vi "Main - 17JuneBackup.vi"() -> ()   [LabVIEW 2018]
uses:
  LoadCellType.ctl
  MotorUnits.ctl
  CalibrationComponentsList.ctl
  CalibrationValuesList.ctl
  CalibrationFileHeaders.ctl
  <vilib>/Analysis/baseanly.llb/Mean (DBL).vi
  1bae0f2e-106e-414f-9c47-dad4a1d3b324.vi
  c2e41f69-c736-4862-8fa9-ab2912e2b40f.vi
  8906c7f1-8855-440d-adf6-1dafab09265a.vi
  e867b6df-3684-438a-bb7f-c804a2c90fcb.vi
  489dc40e-59c5-4e85-922b-f9ff9f858a38.vi
  441b7fa7-1fda-4f0d-8a96-d35181be4240.vi
  76a06f91-e74a-4c68-b1da-59c59035c8f1.vi
  95c3a942-58a8-4429-8ed6-39484f079eb5.vi
  aa792640-a713-44b5-b5bc-ea87e5fc700a.vi
  <vilib>/Utility/file.llb/Write Delimited Spreadsheet (string).vi
  <vilib>/Utility/file.llb/Read Delimited Spreadsheet (string).vi
  <vilib>/FPGAPlugInAG/myRIO-1900/niLvFpga_Open_myRIO-1900.vi
  <vilib>/rvi/interface/common/dynamic/niFpgaDynamicAddResources.vi
  <vilib>/FPGAPlugInAG/Dynamic/niLvFpga_Run_Dynamic.vi
  <vilib>/Utility/error.llb/Error Cluster From Error Code.vi
  <vilib>/rvi/errors/niLvFpgaAdjustHostInterfaceError.vi
  <vilib>/FPGAPlugInAG/Dynamic/niLvFpga_Abort_Dynamic.vi
  <vilib>/FPGAPlugInAG/Dynamic/niLvFpga_Close_Dynamic.vi
  <vilib>/Utility/file.llb/Write Delimited Spreadsheet (DBL).vi
  <vilib>/rvi/interface/nirviOpenFPGA/nirviOpenFPGA.xnode
  FPGA Bitfiles/StandProgram_FPGATarget2_FPGALeftReadout2_EZoqyqWkBrw.lvbitx
  FPGALeftReadout.vi
  <vilib>/rvi/interface/nirviMethod/nirviMethod.xnode
  FPGA Bitfiles/StandProgram_FPGATarget3_FPGARightReadout_3OIjwdsUrXE.lvbitx
  FPGARightReadout.vi
  <vilib>/rvi/interface/nirviReadWriteControl/nirviReadWriteControl.xnode
  <vilib>/rvi/interface/nirviCloseFPGA/nirviCloseFPGA.xnode
  FPGA Bitfiles/StandProgram_FPGATarget_FPGACentreReadou_28m02jle5Aw.lvbitx
  FPGACentreReadout.vi
  NiFpgaLv.dll
  <vilib>/rvi/interface/Simulation/niFpgaSimulationCallBeginRW.vi
  <vilib>/Analysis/NI_AALBase.lvlib
  <userlib>/dxl_x86_c/dxl_x86_c.lvlib
panel:
  out "Torque Timer [s]":dbl
  out "Thrust Timer [s]":dbl
  out "Torque PID out":dbl
  out "Thrust PID out":dbl
  out "Torque error_i":dbl
  out "Torque error_last":dbl
  out "Torque error_d":dbl(graph)
  out "Thrust error_d":dbl(graph)
  out "Thrust error_i":dbl
  out "Thrust error_last":dbl
  in  "PID Min":dbl=60.0 format="%#_13g"
  out "Time under tolerance":dbl
  in  "Torque tolerance [Nm]":dbl=0.01 step=0.001
  in  "Thrust tolerance [g]":dbl=3.0 step=0.1
  out "Torque error [Nm]":dbl
  out "Thrust error [g]":dbl
  in  "Torque Collum":dbl=5.0
  in  "Torque Row":dbl=2.0
  in  "Thrust Collum":dbl=4.0
  in  "Thrust Row":dbl=2.0
  in  "Setlting time [s]":i32=5
  out "Total Torque":dbl(graph)
  out "Total Thrust":dbl(graph)
  in  "PID Max":dbl=1000.0 format="%#_13g"
  in  "kp_m":dbl step=1.0
  in  "ki_m":dbl step=1.0
  in  "kd_m":dbl step=0.1
  in  "kd_t":dbl step=0.1
  in  "ki_t":dbl=0.25 step=0.001
  in  "kp_t":dbl=0.10000000000000003 step=0.1
  out "Closed Loop Left output":dbl
  out "Closed Loop Right output":dbl
  in  "Closed loop":bool
  in  "Total Desired Torque [Nm]":dbl step=0.01
  in  "Total Desired Thrust [g]":dbl step=50.0
  out "Dxl 2 Pos":dbl
  out "Dxl 1 Pos":dbl
  out "Dxl 2 Target Pos":dbl
  out "Timer Dxl 2":dbl
  in  "Collum Dxl 2":dbl=3.0
  in  "Row Dxl 2":dbl=2.0
  out "Dxl 1 Target Pos":dbl
  in  "Row Dxl 1":dbl=2.0
  in  "Collum Dxl 1":dbl=2.0
  out "Timer Dxl 1":dbl
  in  "Collum Left":dbl
  in  "Tare All":bool
  out "Position Raw 1":i32
  out "Position Raw 2":i32
  in  "Row Left":dbl=2.0
  out "PWM Left":dbl(graph)
  out "PWM Left":dbl
  out "Timer Left":dbl
  out "Counts":i32
  out "# of Control Rows":i32=6
  in  "Data  Save Path":string="C:\\Users\\joaos\\Documents\\[PhD]\\Project Omnidirectional Vehicle\\Vanes\\LabView_code\\Experiments Data"
  in  "Control Table Path":string="C:\\Users\\joaos\\Documents\\[PhD]\\Project Omnidirectional Vehicle\\Vanes\\LabView_code\\Control Tables\\Full_system_testing_closed_loop_tune_testing.csv"
  out "PWM Right":dbl
  in  "Record data":bool
  out "PWM Right":dbl(graph)
  out "Timer Right":dbl
  in  "table input switch":bool
  in  "Collum Right":dbl=1.0
  in  "Row Right":dbl=2.0
  out "Table Control":string[][](table)
  out "Centre LC3 Calibration measurement 2":dbl format="%#_13g"
  out "Centre LC2 Calibration measurement 2":dbl format="%#_13g"
  out "Centre LC2 Calibration measurement 1":dbl format="%#_13g"
  out "Centre LC3 Calibration measurement 1":dbl format="%#_13g"
  out "Left LC3 Calibration measurement 2":dbl format="%#_13g"
  out "Left LC2 Calibration measurement 2":dbl format="%#_13g"
  out "Left LC2 Calibration measurement 1":dbl format="%#_13g"
  out "Left LC3 Calibration measurement 1":dbl format="%#_13g"
  out "Right LC3 Calibration measurement 2":dbl format="%#_13g"
  out "Right LC2 Calibration measurement 2":dbl format="%#_13g"
  out "Right LC2 Calibration measurement 1":dbl format="%#_13g"
  out "Right LC3 Calibration measurement 1":dbl format="%#_13g"
  out "LoadCalibrationValues":bool=TRUE
  in  "Values List":T1
  in  "Components List":T2
  in  "Load Calibration Button":bool
  in  "Save Calibration Button":bool
  in  "Motor 2 Operating Mode":u16(ring)=5 caption="Operating Mode" items=["Please Select", "Current Control", "Velocity", "Position", "Extended Position", "Current-based Position Control"]
  out "Current Motor 1 Position":dbl(knob) scale=0.0..360.0
  in  "Motor 1 Operating Mode":u16(ring)=5 caption="Operating Mode" items=["Please Select", "Current Control", "Velocity", "Position", "Extended Position", "Current-based Position Control"]
  out "function return":i32
  in  "Left Stand":enum32{"Main", "Setup"}(tab)
  out "Waveform Chart 2":cluster{dbl, dbl}(graph)
  out "Left Torque":dbl(graph)
  out "Left Motor Frequency":dbl(graph) caption="Motor Speed"
  in  "Left PWM frequency":i16=200 caption="PWM Frequency (Hz)" min=50 max=400
  in  "Left PWM Switch":bool caption="PWM Switch"
  in  "Left PWM pulse width":u32(slide)=1000 caption="PWM Length (us)" min=1000 max=2000 scale=1000.0..2000.0
  out "Left Current":dbl(knob) caption="Current (A)" scale=0.0..90.0
  out "Left Voltage":dbl(knob) caption="Voltage (V)" scale=0.0..60.0
  out "Left Thrust":dbl(graph)
  out "Left LC2":dbl
  out "Left LC3":dbl
  in  "Left Motor Units":T3 caption="Units" items=["RPM", "Hz"]
  in  "Calibrate Torque":bool
  in  "Left LC distance":dbl=0.061 caption="load cell distance (m)"
  in  "Left Calibration arm 2 (m)":dbl=-0.3 caption="Calibration arm 2 (m)"
  in  "Left  Calibration arm 1 (m)":dbl=0.3 caption="Calibration arm 1 (m)"
  out "Left LC1 Reading":i32 caption="Reading"
  in  "Left LC2 and LC3 measure 1":bool
  in  "Left Calibration Weight 1 (g)":dbl=400.74 caption="Calibration Weight 1 (g)"
  in  "Left LC3 Type":T4 caption="Load Cell Type" items=["5kg", "10kg", "50kg"]
  out "Left LC3 zero point":i32 caption="Zero Point"
  in  "Left LC2 and LC3 Tare":bool
  in  "Left LC2 and LC3 measure 2":bool
  in  "Left Calibration Weight 2 (g)":dbl=400.74 caption="Calibration Weight 2 (g)"
  in  "Left LC2 Type":T4 caption="Load Cell Type" items=["5kg", "10kg", "50kg"]
  out "Left LC2 zero point":i32 caption="Zero Point"
  in  "Left LC1 Calibrate":bool
  in  "Left LC1 Calibration Weight (kg)":dbl=400.74 caption="Calibration Weight (kg)"
  in  "Left LC1 Type":T4=1 caption="Load Cell Type" items=["5kg", "10kg", "50kg"]
  out "Left LC1 zero point":i32=34722 caption="Zero Point"
  in  "Left LC1 Tare":bool
  out "Left LC3 Reading":i32 caption="Reading"
  out "Left LC2 Reading":i32 caption="Reading"
  in  "Left Resistance non-Vout (Ohms)":dbl=13.81
  in  "Left Resistance Vout (Ohms)":dbl=1.642
  out "Left Raw Load Cell Readings":cluster{"Data":i32, "Data 2":i32, "Data 3":i32}(graph) caption="Raw Load Cell Readings"
  out "Left LC3 Calibration Constant":dbl format="%#_13g"
  out "Left LC2 Calibration Constant":dbl format="%#_13g"
  out "Left LC1 Calibration Constant":dbl format="%#_13g"
  in  "Centre Stand":enum32{"Main", "Setup"}(tab)
  out "Centre Torque":dbl(graph)
  out "Centre Thrust":dbl(graph)
  out "Centre LC2":dbl
  out "Centre LC3":dbl
  in  "Centre LC distance":dbl=0.055 caption="load cell distance (m)"
  in  "Centre Calibration arm 2 (m)":dbl=0.03 caption="Calibration arm 2 (m)"
  in  "Centre Calibration arm 1 (m)":dbl=-0.032 caption="Calibration arm 1 (m)"
  out "Centre LC1 Reading":i32 caption="Reading"
  in  "Centre  LC2 and LC3 measure 1":bool
  in  "Centre Calibration Weight 2 (g)":dbl=400.74 caption="Calibration Weight 1 (g)"
  in  "Centre LC3 Type":T4=1 caption="Load Cell Type" items=["5kg", "10kg", "50kg"]
  out "Centre LC3 zero point":i32 caption="Zero Point"
  in  "Centre LC3 Tare":bool
  in  "Centre LC2 and LC3 measure 2":bool
  in  "Centre Calibration Weight 1 (g)":dbl=400.74 caption="Calibration Weight 2 (g)"
  in  "Centre LC2 Type":T4=1 caption="Load Cell Type" items=["5kg", "10kg", "50kg"]
  out "Centre LC2 zero point":i32 caption="Zero Point"
  in  "Calibrate Torque":bool
  in  "Centre LC1 Calibrate":bool
  in  "Centre LC1 Calibration Weight (g)":dbl=400.74 caption="Calibration Weight (g)"
  in  "Centre LC1 Type":T4=1 caption="Load Cell Type" items=["5kg", "10kg", "50kg"]
  out "Centre LC1 zero point":i32=34722 caption="Zero Point"
  in  "Centre LC1 Tare":bool
  out "Centre LC3 Reading":i32 caption="Reading"
  out "Centre LC2 Reading":i32 caption="Reading"
  out "Centre Raw Load Cell Readings":cluster{"Data":i32, "Data 2":i32, "Data 3":i32}(graph) caption="Raw Load Cell Readings"
  out "Centre LC3 Calibration Constant":dbl format="%#_13g"
  out "Centre LC2 Calibration Constant":dbl format="%#_13g"
  out "Centre LC1 Calibration Constant":dbl format="%#_13g"
  out "StopLoops":bool
  in  "Program Stop":bool
  out "Current Motor 2 Position":dbl(knob) scale=0.0..360.0
  in  "Target Motor 2 Position":dbl(slide) scale=-90.0..90.0
  in  "Target Motor 1 Position":dbl(slide) scale=-90.0..90.0
  in  "Right Stand":enum32{"Main", "Setup"}(tab)
  out "Waveform Chart":cluster{dbl, dbl}(graph)
  out "Right Motor Frequency":dbl(graph) caption="Motor Speed"
  in  "Right PWM frequency":i16=200 caption="PWM Frequency (Hz)" min=50 max=400
  in  "Right PWM Switch":bool caption="PWM Switch"
  in  "Right PWM Slide":u32(slide)=1000 caption="PWM Length (us)" min=1000 max=2000 scale=1000.0..2000.0
  out "Right Current":dbl(knob) caption="Current (A)" scale=0.0..90.0
  out "Right Voltage":dbl(knob) caption="Voltage (V)" scale=0.0..60.0
  out "Right Thrust":dbl(graph)
  out "Right LC2":dbl
  out "Right LC3":dbl
  in  "Right Motor Units":T3 caption="Units" items=["RPM", "Hz"]
  out "Right Torque":dbl(graph)
  in  "Right LC distance":dbl=0.062 caption="load cell distance (m)"
  in  "Toque calibrate":bool
  in  "Right LC2 and LC3 measure 2":bool
  in  "Right Calibration arm 2 (m)":dbl=0.3 caption="Calibration arm 2 (m)"
  in  "Right Resistance Vout (Ohms)":dbl=1.642
  in  "Right Resistance non-Vout (Ohms)":dbl=13.81
  in  "Right Calibration arm 1 (m)":dbl=-0.3 caption="Calibration arm 1 (m)"
  out "Right LC1 Reading":i32 caption="Reading"
  in  "Right Calibration Weight 1 (g)":dbl=400.74 caption="Calibration Weight 1 (g)"
  in  "Right LC3 Type":T4 caption="Load Cell Type" items=["5kg", "10kg", "50kg"]
  out "Right LC3 zero point":i32 caption="Zero Point"
  in  "Right LC2 and LC3 measure 1":bool
  in  "Right Calibration Weight 2 (g)":dbl=400.74 caption="Calibration Weight 2 (g)"
  in  "Right LC2 Type":T4 caption="Load Cell Type" items=["5kg", "10kg", "50kg"]
  out "Right LC2 zero point":i32 caption="Zero Point"
  in  "Right LC2 and LC3 Tare":bool
  in  "Right LC1 Calibrate":bool
  in  "Right LC1 Calibration Weight (kg)":dbl=400.74 caption="Calibration Weight (g)"
  in  "Right LC1 Type":T4=1 caption="Load Cell Type" items=["5kg", "10kg", "50kg"]
  out "Right LC1 zero point":i32=34722 caption="Zero Point"
  in  "Right LC1 Tare":bool
  out "Right LC3 Reading":i32 caption="Reading"
  out "Right LC2 Reading":i32 caption="Reading"
  out "Right Raw Load Cell Readings":cluster{"Data":i32, "Data 2":i32, "Data 3":i32}(graph) caption="Raw Load Cell Readings"
  out "Right LC1 Calibration Constant":dbl format="%#_13g"
  out "Right LC2 Calibration Constant":dbl format="%#_13g"
  out "Right LC3 Calibration Constant":dbl format="%#_13g"
  # "Automatic Control"
  # "For Closed-loop"
  # "Thrust PID Gains"
  # "Torque PID Gains"
  # "Left Stand"
  # "Right Stand"
  # "Centre Stand"
  # "Motor 1 Control"
  # "Motor 2 Control"
  # "Position Degrees"
  # "Position  Degrees"
  # "Set position"
  # "Set position"
  # "Load Cell 1"
  # "Voltmeter"
  # "Load Cell 3"
  # "Load Cell 2"
  # "Load Cell 1"
  # "Load Cell 3"
  # "Load Cell 2"
  # "Load Cell 1"
  # "Voltmeter"
  # "Load Cell 3"
  # "Load Cell 2"
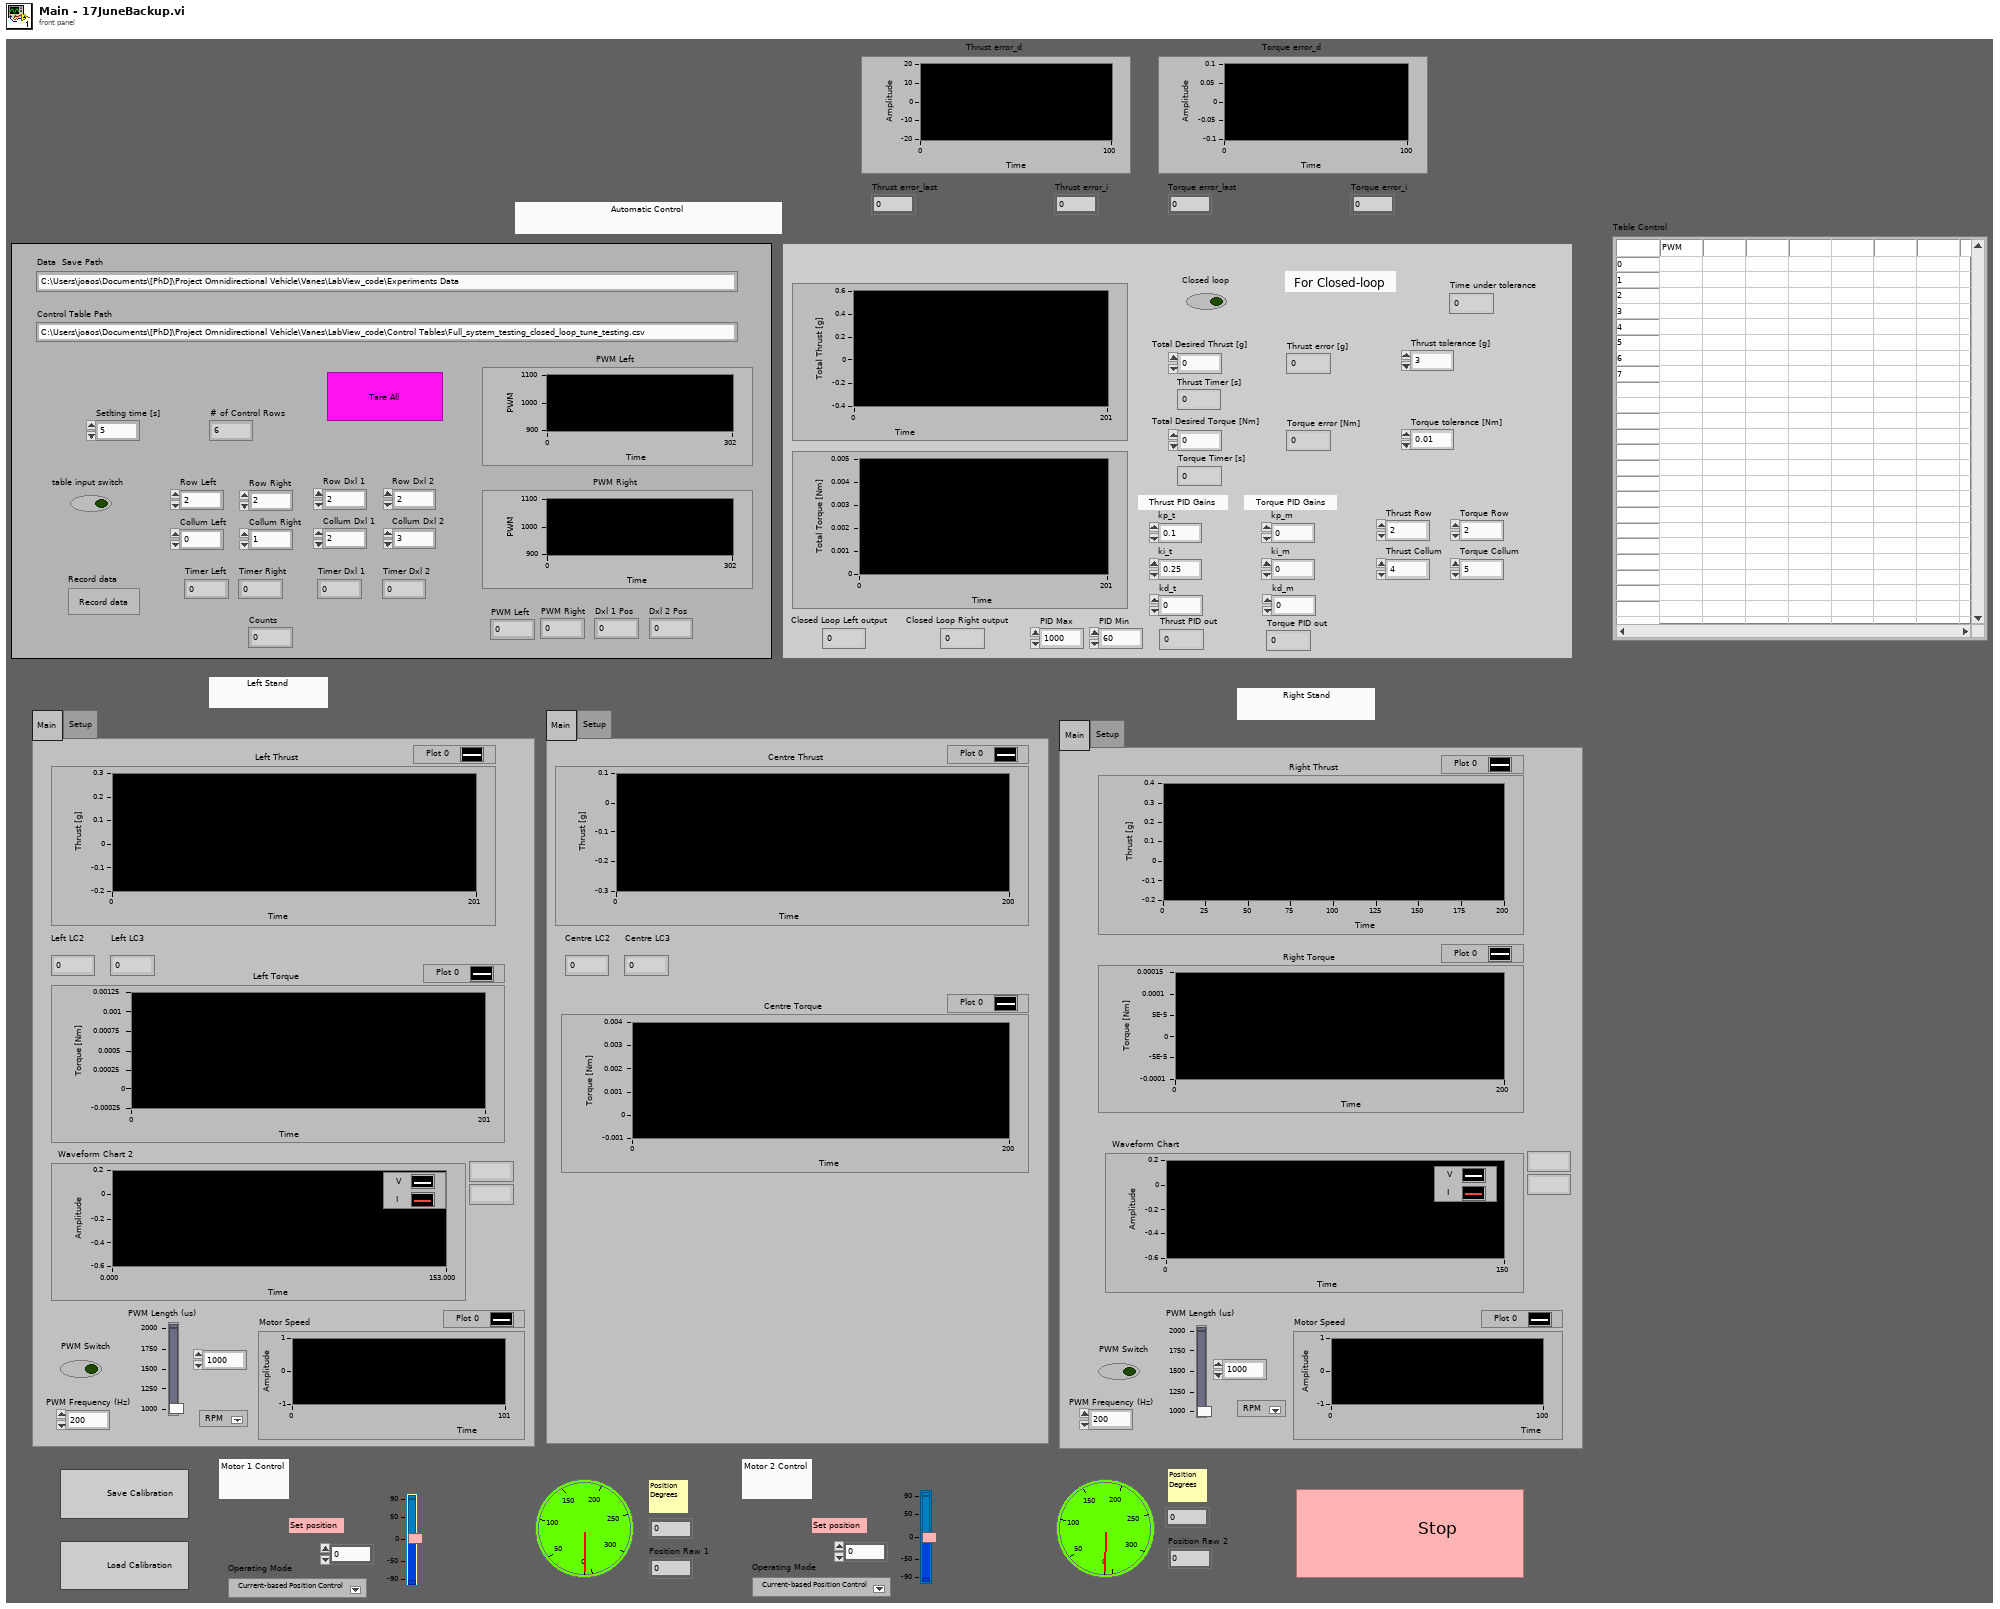
[diagram p1: front panel]
types:
  T1 = typedef "CalibrationValuesList.ctl" = string[]
  T2 = typedef "CalibrationComponentsList.ctl" = string[]
  T3 = typedef "MotorUnits.ctl" = u16
  T4 = typedef "LoadCellType.ctl" = u16
  T5 = typedef "CalibrationFileHeaders.ctl" = string[]
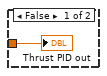
[diagram p4: hidden frame]
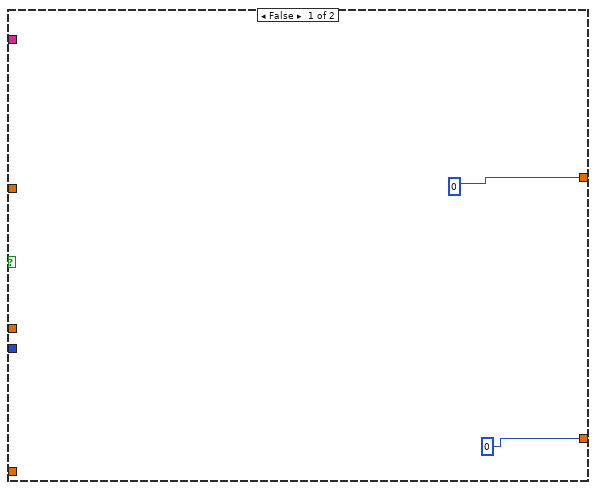
[diagram p8: hidden frame]
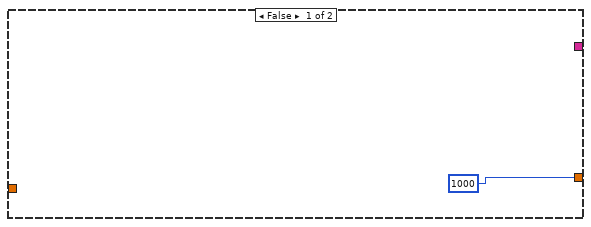
[diagram p12: hidden frame]
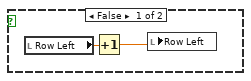
[diagram p14: hidden frame]
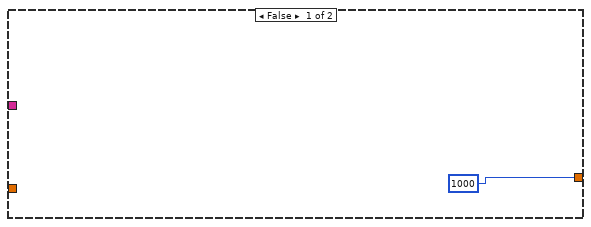
[diagram p15: hidden frame]
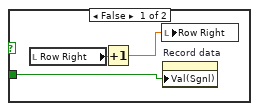
[diagram p17: hidden frame]
diagram:
  (unwired) T5 ["Component", "Value"] ("Headers")
  n1 = stacked-sequence {
    tunnel: [_ _ w64] -> w23
    tunnel: [_ _ w61] -> w20
    tunnel: [_ _ w60] -> w19
    tunnel: [_ _ w57] -> w18
    tunnel: [_ _ w54] -> w17
    tunnel: [_ _ w53] -> w16
    tunnel: [_ _ w50] -> w15
    tunnel: [_ _ w45] -> w14
    tunnel: [w42 _ _] -> w13
    frame #0 {
      n2 = property on="LoadCalibrationValues" class="Bool (strict)"("Val(Sgnl)"=TRUE ("Value (Signaling)")) -> (error out=w42:errorcluster)  [unwired: 2 in, 1 out]
    }
    frame #1 {
      n3 = Wait (ms)(milliseconds to wait=u32 100) -> ()  [unwired: 1 out]
    }
    frame #2 {
      n4 = xnode "Open FPGA VI Reference"() -> ("FPGA VI Reference Out"=w65:refnum<k20>)  [unwired: 2 in, 1 out]
      n5 = invoke on="Left PWM pulse width" class="Slide (strict)" method="Reinit To Default"() -> (error out=w57:errorcluster)  [unwired: 3 in, 2 out]
      n6 = xnode "Invoke Method"("FPGA VI Reference In"=w65) -> ("FPGA VI Reference Out"=w64:refnum<k20>)  [unwired: 2 in, 1 out]
      n7 = Initialize Array(0.0 ("element"), 10 ("dimension size")) -> (w54:dbl[])
      n8 = Initialize Array(0.0 ("element"), 10 ("dimension size")) -> (w53:dbl[])
      n9 = Initialize Array(0.0 ("element"), 10 ("dimension size")) -> (w60:dbl[])
      n10 = Initialize Array(0.0 ("element"), 10 ("dimension size")) -> (w45:dbl[])
      n11 = Initialize Array(0.0 ("element"), 10 ("dimension size")) -> (w61:dbl[])
      n12 = Initialize Array(0.0 ("element"), 10 ("dimension size")) -> (w50:dbl[])
    }
  }
  n13 = while {
    tunnel: w23 -> [w81]
    tunnel: [w80] -> w21
    shift-right: [w77] -> _
    shift-left: w20 -> [w78]
    shift-right: [w74] -> _
    shift-left: w19 -> [w75]
    tunnel: w18 -> [_]
    shift-right: [w72] -> _
    shift-left: w17 -> [w73]
    shift-right: [w70] -> _
    shift-left: w16 -> [w71]
    shift-right: [w68] -> _
    shift-left: w15 -> [w69]
    shift-right: [w67] -> _
    shift-left: w14 -> [w66]
    stop <- w82 stop-if-true
    # "Left Stand"
    n14 = case shown="\"Main\", Default" "Left Stand" {
      tunnel: w81 -> [w179 w231]
      tunnel: [w132 w226] -> w80
      tunnel: w78 -> [w171 w222]
      tunnel: [w94 w220] -> w77
      tunnel: w75 -> [w156 w218]
      tunnel: [w155 w218] -> w74
      tunnel: w73 -> [w140 w217]
      tunnel: [w135 w217] -> w72
      tunnel: w71 -> [w127 w213]
      tunnel: [w124 w213] -> w70
      tunnel: w69 -> [w119 w209]
      tunnel: [w93 w207] -> w68
      tunnel: w66 -> [w109 w205]
      tunnel: [w92 w206] -> w67
      frame "Main", Default {
        n15 = xnode "Read/Write Control"("FPGA VI Reference In"=w179) -> ("FPGA VI Reference Out"=w178:refnum<k20>, "RawVoltage"=w154:i16)  [unwired: 1 in, 1 out]
        n16 = Delete From Array(array=w119, length=1, index=0) -> (array with subset deleted=w120:dbl[])  [unwired: 1 out]
        n17 = Delete From Array(array=w109, length=1, index=0) -> (array with subset deleted=w113:dbl[])  [unwired: 1 out]
        n18 = Delete From Array(array=w140, length=1, index=0) -> (array with subset deleted=w139:dbl[])  [unwired: 1 out]
        n19 = Delete From Array(array=w156, length=1, index=0) -> (array with subset deleted=w162:dbl[])  [unwired: 1 out]
        n20 = Delete From Array(array=w171, length=1, index=0) -> (array with subset deleted=w174:dbl[])  [unwired: 1 out]
        n21 = xnode "Read/Write Control"("FPGA VI Reference In"=w178) -> ("FPGA VI Reference Out"=w177:refnum<k20>, "RawCurrent"=w136:u16)  [unwired: 1 in, 1 out]
        n22 = Build Array (concatenate)(w139, w136) -> (w135:dbl[])
        n23 = Build Array (concatenate)(w162, w154) -> (w155:dbl[])
        n24 = call-poly <vilib>:"Mean.vi"("X"=w135) -> ("mean"=w134:dbl)  [unwired: 1 out]
        n25 = call-poly <vilib>:"Mean.vi"("X"=w155) -> ("mean"=w160:dbl)  [unwired: 1 out]
        n26 = Divide(x=i16 20, y=i16 4096) -> (x/y=w161:dbl)
        n27 = Multiply(x=w160, y=w161) -> (x*y=w158:dbl)
        n28 = xnode "Read/Write Control"("FPGA VI Reference In"=w177) -> ("FPGA VI Reference Out"=w176:refnum<k20>, "Data"=w167:i32)  [unwired: 1 in, 1 out]
        n29 = Build Array (concatenate)(w174, w167) -> (w94:dbl[])
        n30 = call-poly <vilib>:"Mean.vi"("X"=w94) -> ("mean"=w87:dbl)  [unwired: 1 out]
        n31 = property on="Left LC1 zero point" class="DigNum (strict)"() -> ("Value"=w168:i32)  [unwired: 2 in, 2 out]
        n32 = Add(x="Left Resistance Vout (Ohms)", y="Left Resistance non-Vout (Ohms)") -> (x+y=w153:dbl)
        n33 = property on="Left LC2 zero point" class="DigNum (strict)"() -> ("Value"=w117:i32)  [unwired: 2 in, 2 out]
        n34 = Subtract(x=w87, y=w168) -> (x-y=w169:dbl)
        n35 = property on="Left LC1 Calibration Constant" class="DigNum (strict)"() -> ("Value"=w170:dbl)  [unwired: 2 in, 2 out]
        n36 = property on="Left LC3 zero point" class="DigNum (strict)"() -> ("Value"=w115:i32)  [unwired: 2 in, 2 out]
        n37 = property on="Left LC2 Calibration Constant" class="DigNum (strict)"() -> ("Value"=w118:dbl)  [unwired: 2 in, 2 out]
        n38 = xnode "Read/Write Control"("FPGA VI Reference In"=w176) -> ("FPGA VI Reference Out"=w175:refnum<k20>, "Data 2"=w116:i32)  [unwired: 1 in, 1 out]
        n39 = Build Array (concatenate)(w120, w116) -> (w93:dbl[])
        n40 = call-poly <vilib>:"Mean.vi"("X"=w93) -> ("mean"=w86:dbl)  [unwired: 1 out]
        n41 = Subtract(x=w86, y=w117) -> (x-y=w123:dbl)
        n42 = property on="Left LC3 Calibration Constant" class="DigNum (strict)"() -> ("Value"=w114:dbl)  [unwired: 2 in, 2 out]
        n43 = Divide(x=w153, y="Left Resistance Vout (Ohms)") -> (x/y=w157:dbl)
        n44 = Multiply(x=w157, y=w158) -> (x*y=w91:dbl)
        "Left Voltage" <- w91
        n45 = Divide(x=i16 5, y=i16 4096) -> (x/y=w149:dbl)
        n46 = Multiply(x=w170, y=w169) -> (x*y=→"Left Thrust":dbl)
        n47 = Multiply(x=w118, y=w123) -> (x*y=w98:dbl)
        "Left LC2" <- w98
        n48 = Multiply(x=w134, y=w149) -> (x*y=w141:dbl)
        n49 = Divide(x=i16 90 ("y"), y=3.3 ("x")) -> (x/y=w148:dbl)
        n50 = xnode "Read/Write Control"("FPGA VI Reference In"=w175) -> ("FPGA VI Reference Out"=w147:refnum<k20>, "Data 3"=w108:i32)  [unwired: 1 in, 1 out]
        n51 = Build Array (concatenate)(w113, w108) -> (w92:dbl[])
        n52 = call-poly <vilib>:"Mean.vi"("X"=w92) -> ("mean"=w85:dbl)  [unwired: 1 out]
        n53 = Subtract(x=w85, y=w115) -> (x-y=w110:dbl)
        n54 = Multiply(x=w114, y=w110) -> (x*y=w97:dbl)
        "Left LC3" <- w97
        n55 = Multiply(x=w141, y=w148) -> (x*y=w90:dbl)
        "Left Current" <- w90
        n56 = local read "PWM Left"() -> (w88:dbl)
        n57 = Add(x=w98, y=w97) -> (x+y=w104:dbl)
        n58 = property on="Left LC distance" class="DigNum (strict)"() -> ("Value"=w96:dbl)  [unwired: 2 in, 2 out]
        n59 = local read "Tare All"() -> (w84:bool)
        n60 = Divide(x=w96, y=2) -> (x/y=w103:dbl)
        n61 = xnode "Read/Write Control"("FPGA VI Reference In"=w147, "Pulse Width (us)"=w88) -> ("FPGA VI Reference Out"=w146:refnum<k20>)  [unwired: 1 in, 1 out]
        n62 = Bundle(cluster=cluster{dbl, dbl} {0.0, 0.0}, w91, w90) -> (→"Waveform Chart 2":cluster{dbl, dbl})
        n63 = case shown="True" w84 {
          tunnel: [_ w184] -> _
          tunnel: w87 -> [_ w183]
          frame False {
          }
          frame True {
            n64 = property on="Left LC1 zero point" class="DigNum (strict)"("Val(Sgnl)"=w183) -> (error out=w184:errorcluster)  [unwired: 2 in, 1 out]
          }
        }
        n65 = Multiply(x=w103, y=w104) -> (x*y=w102:dbl)
        n66 = Divide(x=9.81, y=1000) -> (x/y=w99:dbl)
        n67 = Multiply(x=w102, y=w99) -> (x*y=→"Left Torque":dbl)
        n68 = xnode "Read/Write Control"("FPGA VI Reference In"=w146, "Frequency"="Left PWM frequency") -> ("FPGA VI Reference Out"=w145:refnum<k20>)  [unwired: 1 in, 1 out]
        n69 = case shown="True" w84 {
          tunnel: [_ w182] -> _
          tunnel: w86 -> [_ w181]
          tunnel: w85 -> [_ w180]
          frame False {
          }
          frame True {
            n70 = property on="Left LC3 zero point" class="DigNum (strict)"("Val(Sgnl)"=w180) -> ()  [unwired: 2 in, 2 out]
            n71 = property on="Left LC2 zero point" class="DigNum (strict)"("Val(Sgnl)"=w181) -> (error out=w182:errorcluster)  [unwired: 2 in, 1 out]
          }
        }
        n72 = xnode "Read/Write Control"("FPGA VI Reference In"=w145, "PWM Switch"="Left PWM Switch") -> ("FPGA VI Reference Out"=w144:refnum<k20>)  [unwired: 1 in, 1 out]
        n73 = xnode "Read/Write Control"("FPGA VI Reference In"=w144) -> ("FPGA VI Reference Out"=w132:refnum<k20>, "Rotor Speed (Hz)"=w131:sgl)  [unwired: 1 in, 1 out]
        n74 = case shown="True" "Left PWM Switch" {
          tunnel: [0.0 ("Motor Frequency") w187] -> w126
          tunnel: w131 -> [_ w186]
          frame False {
          }
          frame True {
            w193 = T3 1 items=["RPM", "Hz"] ("Right Motor Units")
            n75 = Equal?(x="Left Motor Units", y=w193) -> (x = y?=w192:bool)
            n76 = Select(t=1.0, s=w192, f=60.0) -> (s? t:f=w188:dbl)
            n77 = Multiply(x=w188, y=w186) -> (x*y=w187:dbl)
          }
        }
        n78 = Delete From Array(array=w127, length=1, index=0) -> (array with subset deleted=w128:dbl[])  [unwired: 1 out]
        n79 = Build Array (concatenate)(w128, w126) -> (w124:dbl[])
        n80 = call-poly <vilib>:"Mean.vi"("X"=w124) -> ("mean"=→"Left Motor Frequency":dbl)  [unwired: 1 out]
      }
      frame "Setup" {
        n81 = xnode "Read/Write Control"("FPGA VI Reference In"=w231) -> ("FPGA VI Reference Out"=w230:refnum<k20>)  [unwired: 1 in, 2 out]
        n82 = Delete From Array(array=w222, length=1, index=0) -> (array with subset deleted=w221:dbl[])  [unwired: 1 out]
        n83 = Delete From Array(array=w205, length=1, index=0) -> (array with subset deleted=w202:dbl[])  [unwired: 1 out]
        n84 = Delete From Array(array=w209, length=1, index=0) -> (array with subset deleted=w212:dbl[])  [unwired: 1 out]
        n85 = xnode "Read/Write Control"("FPGA VI Reference In"=w230) -> ("FPGA VI Reference Out"=w229:refnum<k20>)  [unwired: 1 in, 2 out]
        n86 = xnode "Read/Write Control"("FPGA VI Reference In"=w229) -> ("FPGA VI Reference Out"=w228:refnum<k20>, "Data"=w216:i32)  [unwired: 1 in, 1 out]
        "Left LC1 Reading" <- w216
        n87 = Build Array (concatenate)(w221, w216) -> (w220:dbl[])
        n88 = call-poly <vilib>:"Mean.vi"("X"=w220) -> ("mean"=w219:dbl)  [unwired: 1 out]
        n89 = xnode "Read/Write Control"("FPGA VI Reference In"=w228) -> ("FPGA VI Reference Out"=w227:refnum<k20>, "Data 2"=w208:i32)  [unwired: 1 in, 1 out]
        "Left LC2 Reading" <- w208
        n90 = Build Array (concatenate)(w212, w208) -> (w207:dbl[])
        n91 = call-poly <vilib>:"Mean.vi"("X"=w207) -> ("mean"=w199:dbl)  [unwired: 1 out]
        n92 = case shown="True" "Left LC1 Tare" {
          tunnel: w219 -> [_ w286]
          tunnel: [FALSE TRUE] -> _
          tunnel: [_ w284] -> _
          frame False {
          }
          frame True {
            n93 = property on="Left LC1 zero point" class="DigNum (strict)"("Val(Sgnl)"=w286) -> (error out=w284:errorcluster)  [unwired: 2 in, 1 out]
          }
        }
        n94 = case shown="True" "Left LC1 Calibrate" {
          tunnel: w219 -> [_ w282]
          frame False {
          }
          frame True {
            n95 = local read "Left LC1 zero point"() -> (w281:i32)
            n96 = Subtract(x=w282, y=w281) -> (x-y=w280:dbl)
            n97 = Divide(x="Left LC1 Calibration Weight (kg)", y=w280) -> (x/y=→"Left LC1 Calibration Constant":dbl)
          }
        }
        n98 = xnode "Read/Write Control"("FPGA VI Reference In"=w227) -> ("FPGA VI Reference Out"=w226:refnum<k20>, "Data 3"=w201:i32)  [unwired: 1 in, 1 out]
        "Left LC3 Reading" <- w201
        n99 = Build Array (concatenate)(w202, w201) -> (w206:dbl[])
        n100 = call-poly <vilib>:"Mean.vi"("X"=w206) -> ("mean"=w198:dbl)  [unwired: 1 out]
        n101 = case shown="True" "Left LC2 and LC3 measure 2" {
          tunnel: w198 -> [_ w265]
          tunnel: w199 -> [_ w266]
          frame False {
          }
          frame True {
            n102 = local read "Left LC2 zero point"() -> (w268:i32)
            n103 = local read "Left LC3 zero point"() -> (w267:i32)
            n104 = Subtract(x=w266, y=w268) -> (x-y=→"Left LC2 Calibration measurement 2":dbl)
            n105 = Subtract(x=w265, y=w267) -> (x-y=→"Left LC3 Calibration measurement 2":dbl)
          }
        }
        n106 = case shown="True" "Left LC2 and LC3 measure 1" {
          tunnel: w198 -> [_ w271]
          tunnel: w199 -> [_ w272]
          frame False {
          }
          frame True {
            n107 = local read "Left LC2 zero point"() -> (w274:i32)
            n108 = local read "Left LC3 zero point"() -> (w273:i32)
            n109 = Subtract(x=w272, y=w274) -> (x-y=→"Left LC2 Calibration measurement 1":dbl)
            n110 = Subtract(x=w271, y=w273) -> (x-y=→"Left LC3 Calibration measurement 1":dbl)
          }
        }
        n111 = case shown="True" "Left LC2 and LC3 Tare" {
          tunnel: w199 -> [_ w277]
          tunnel: [_ w276] -> _
          tunnel: w198 -> [_ w275]
          frame False {
          }
          frame True {
            n112 = property on="Left LC2 zero point" class="DigNum (strict)"("Val(Sgnl)"=w277) -> (error out=w276:errorcluster)  [unwired: 2 in, 1 out]
            n113 = property on="Left LC3 zero point" class="DigNum (strict)"("Val(Sgnl)"=w275) -> ()  [unwired: 2 in, 2 out]
          }
        }
        n114 = case shown="True" "Calibrate Torque" {
          frame False {
          }
          frame True {
            n115 = local read "Left LC3 Calibration measurement 2"() -> (w238:dbl)
            n116 = local read "Left LC2 Calibration measurement 1"() -> (w259:dbl)
            n117 = local read "Left LC3 Calibration measurement 1"() -> (w261:dbl)
            n118 = local read "Left LC2 Calibration measurement 2"() -> (w233:dbl)
            n119 = local read "Left LC distance"() -> (w243:dbl)
            n120 = Multiply(x="Left Calibration Weight 2 (g)", y=2) -> (x*y=w246:dbl)
            n121 = Multiply(x="Left Calibration Weight 1 (g)", y=2) -> (x*y=w253:dbl)
            n122 = Multiply(x=w246, y="Left Calibration arm 2 (m)") -> (x*y=w244:dbl)
            n123 = Multiply(x=w253, y="Left  Calibration arm 1 (m)") -> (x*y=w251:dbl)
            n124 = Divide(x=w244, y=w243) -> (x/y=w242:dbl)
            n125 = Divide(x=w251, y="Left LC distance") -> (x/y=w249:dbl)
            n126 = Divide(x=w261, y=w238) -> (x/y=w241:dbl)
            n127 = Multiply(x=w241, y=w242) -> (x*y=w240:dbl)
            n128 = Subtract(x=w249, y=w240) -> (x-y=w239:dbl)
            n129 = Multiply(x=w241, y=w233) -> (x*y=w260:dbl)
            n130 = Divide(x=1, y=w238) -> (x/y=w236:dbl)
            n131 = Subtract(x=w259, y=w260) -> (x-y=w257:dbl)
            n132 = Divide(x=1, y=w257) -> (x/y=w256:dbl)
            n133 = Multiply(x=w256, y=w239) -> (x*y=w232:dbl)
            "Left LC2 Calibration Constant" <- w232
            n134 = Multiply(x=w233, y=w232) -> (x*y=w234:dbl)
            n135 = Subtract(x=w242, y=w234) -> (x-y=w235:dbl)
            n136 = Multiply(x=w235, y=w236) -> (x*y=→"Left LC3 Calibration Constant":dbl)
          }
        }
        n137 = Bundle(cluster=cluster{"Data":i32, "Data 2":i32, "Data 3":i32} {"Data"=0, "Data 2"=0, "Data 3"=0}, "Data"=w216, "Data 2"=w208, "Data 3"=w201) -> (→"Left Raw Load Cell Readings":cluster{"Data":i32, "Data 2":i32, "Data 3":i32})
      }
    }
    n138 = Wait (ms)(milliseconds to wait=u32 5) -> ()  [unwired: 1 out]
    n139 = local read "StopLoops"() -> (w82:bool)
  }
  n140 = invoke on="StopLoops" class="Bool (strict)" method="Reinit To Default"() -> (error out=w40:errorcluster)  [unwired: 3 in, 2 out]
  n141 = invoke on="Program Stop" class="Bool (strict)" method="Reinit To Default"() -> (error out=w41:errorcluster)  [unwired: 3 in, 2 out]
  n142 = while {
    tunnel: w41 -> [_]
    tunnel: w40 -> [_]
    stop <- w287 stop-if-true
    n143 = event shown="[3] \"Load Calibration Button\", \"LoadCalibrationValues\": Value Change" {
      selector: _ -> [_ _ _ _]
      dyn-events: _ -> [_ _ _ _]
      timeout: _ -> [_ _ _ _]
      tunnel: [_ w289 _ _] -> w287
      event Timeout {
        n144 = event-data() -> ()  [unwired: 1 in, 3 out]
      }
      event "Program Stop": Value Change {
        w289 = TRUE
        n145 = event-data() -> ()  [unwired: 1 in, 6 out]
        "StopLoops" <- w289
      }
      event "Save Calibration Button": Value Change {
        n146 = event-data() -> ("NewVal"=w290:bool)  [unwired: 1 in, 5 out]
        n147 = case shown="True" w290 {
          frame False {
          }
          frame True {
            w323 = i16 12 ("precision (6)")
            w327 = i16 12 ("precision (6)")
            n148 = property on="Left LC2 zero point" class="DigNum (strict)"() -> ("Value"=w315:i32)  [unwired: 2 in, 2 out]
            n149 = property on="Left LC3 zero point" class="DigNum (strict)"() -> ("Value"=w316:i32)  [unwired: 2 in, 2 out]
            n150 = property on="Left LC1 zero point" class="DigNum (strict)"() -> ("Value"=w314:i32)  [unwired: 2 in, 2 out]
            n151 = property on="Left LC3 Calibration Constant" class="DigNum (strict)"() -> ("Value"=w334:dbl)  [unwired: 2 in, 2 out]
            n152 = property on="Left LC2 Calibration Constant" class="DigNum (strict)"() -> ("Value"=w335:dbl)  [unwired: 2 in, 2 out]
            n153 = property on="Left LC1 Calibration Constant" class="DigNum (strict)"() -> ("Value"=w336:dbl)  [unwired: 2 in, 2 out]
            n154 = Number To Fractional String(number=w315, precision (6)=w323) -> (F-format string=w311:string)  [unwired: 2 in]
            n155 = Number To Fractional String(number=w316, precision (6)=w323) -> (F-format string=w309:string)  [unwired: 2 in]
            n156 = Number To Fractional String(number=w335, precision (6)=w327) -> (F-format string=w310:string)  [unwired: 2 in]
            n157 = Number To Fractional String(number=w314, precision (6)=w323) -> (F-format string=w313:string)  [unwired: 2 in]
            n158 = Number To Fractional String(number=w334, precision (6)=w327) -> (F-format string=w308:string)  [unwired: 2 in]
            n159 = Number To Fractional String(number=w336, precision (6)=w327) -> (F-format string=w312:string)  [unwired: 2 in]
            n160 = property on="Centre LC3 zero point" class="DigNum (strict)"() -> ("Value"=w317:i32)  [unwired: 2 in, 2 out]
            n161 = property on="Centre LC2 zero point" class="DigNum (strict)"() -> ("Value"=w318:i32)  [unwired: 2 in, 2 out]
            n162 = property on="Centre LC1 zero point" class="DigNum (strict)"() -> ("Value"=w319:i32)  [unwired: 2 in, 2 out]
            n163 = property on="Centre LC3 Calibration Constant" class="DigNum (strict)"() -> ("Value"=w333:dbl)  [unwired: 2 in, 2 out]
            n164 = property on="Centre LC2 Calibration Constant" class="DigNum (strict)"() -> ("Value"=w332:dbl)  [unwired: 2 in, 2 out]
            n165 = property on="Centre LC1 Calibration Constant" class="DigNum (strict)"() -> ("Value"=w331:dbl)  [unwired: 2 in, 2 out]
            n166 = Number To Fractional String(number=w318, precision (6)=w323) -> (F-format string=w305:string)  [unwired: 2 in]
            n167 = Number To Fractional String(number=w317, precision (6)=w323) -> (F-format string=w303:string)  [unwired: 2 in]
            n168 = Number To Fractional String(number=w332, precision (6)=w327) -> (F-format string=w304:string)  [unwired: 2 in]
            n169 = Number To Fractional String(number=w319, precision (6)=w323) -> (F-format string=w307:string)  [unwired: 2 in]
            n170 = Number To Fractional String(number=w333, precision (6)=w327) -> (F-format string=w302:string)  [unwired: 2 in]
            n171 = Number To Fractional String(number=w331, precision (6)=w327) -> (F-format string=w306:string)  [unwired: 2 in]
            n172 = property on="Right LC3 zero point" class="DigNum (strict)"() -> ("Value"=w320:i32)  [unwired: 2 in, 2 out]
            n173 = property on="Right LC2 zero point" class="DigNum (strict)"() -> ("Value"=w321:i32)  [unwired: 2 in, 2 out]
            n174 = property on="Right LC1 zero point" class="DigNum (strict)"() -> ("Value"=w322:i32)  [unwired: 2 in, 2 out]
            n175 = property on="Right LC3 Calibration Constant" class="DigNum (strict)"() -> ("Value"=w330:dbl)  [unwired: 2 in, 2 out]
            n176 = property on="Right LC2 Calibration Constant" class="DigNum (strict)"() -> ("Value"=w329:dbl)  [unwired: 2 in, 2 out]
            n177 = property on="Right LC1 Calibration Constant" class="DigNum (strict)"() -> ("Value"=w328:dbl)  [unwired: 2 in, 2 out]
            n178 = Number To Fractional String(number=w321, precision (6)=w323) -> (F-format string=w299:string)  [unwired: 2 in]
            n179 = Number To Fractional String(number=w320, precision (6)=w323) -> (F-format string=w297:string)  [unwired: 2 in]
            n180 = Number To Fractional String(number=w329, precision (6)=w327) -> (F-format string=w298:string)  [unwired: 2 in]
            n181 = Number To Fractional String(number=w322, precision (6)=w323) -> (F-format string=w301:string)  [unwired: 2 in]
            n182 = Number To Fractional String(number=w330, precision (6)=w327) -> (F-format string=w296:string)  [unwired: 2 in]
            n183 = Number To Fractional String(number=w328, precision (6)=w327) -> (F-format string=w300:string)  [unwired: 2 in]
            n184 = Build Array(w313, w312, w311, w310, w309, w308, w307, w306, w305, w304, w303, w302, w301, w300, w299, w298, w297, w296) -> (w295:string[])
            n185 = Build Array(string[] ["Left LC1 Zero Point", "Left LC1 Calibration Constant", "Left LC2 Zero Point", "Left LC2 Calibration Constant", "Left LC3 Zero Point", "Left LC3 Calibration Constant", "Centre LC1 Zero Point", "Centre LC1 Calibration Constant", "Centre LC2 Zero Point", "Centre LC2 Calibration Constant", "Centre LC3 Zero Point", "Centre LC3 Calibration Constant", "Right LC1 Zero Point", "Right LC1 Calibration Constant", "Right LC2 Zero Point", "Right LC2 Calibration Constant", "Right LC3 Zero Point", "Right LC3 Calibration Constant"] ("Components List"), w295) -> (w294:string[][])
            n186 = Current VI's Path() -> (path=w293:path)
            n187 = Strip Path(path=w293) -> (stripped path=w292:path)  [unwired: 1 out]
            n188 = Build Path(base path=w292, name or relative path="CalibrationValues.csv") -> (appended path=w325:path)
            n189 = call-poly <vilib>:"Write Delimited Spreadsheet.vi"("file path (dialog if empty)"=w325, "2D data"=w294, "delimiter (\\t)"="," ("delimiter (\\t)")) -> ()  [unwired: 11 in, 2 out]
          }
        }
      }
      event "Load Calibration Button", "LoadCalibrationValues": Value Change {
        n190 = event-data() -> ("NewVal"=w337:bool)  [unwired: 1 in, 5 out]
        n191 = case shown="True" w337 {
          frame False {
          }
          frame True {
            n192 = Current VI's Path() -> (path=w345:path)
            n193 = Strip Path(path=w345) -> (stripped path=w346:path)  [unwired: 1 out]
            n194 = Build Path(base path=w346, name or relative path="CalibrationValues.csv") -> (appended path=w343:path)
            n195 = call-poly <vilib>:"Read Delimited Spreadsheet.vi"("file path (dialog if empty)"=w343, "delimiter (\\t)"="," ("delimiter (\\t)")) -> ("all rows"=w341:string[][])  [unwired: 8 in, 5 out]
            n196 = Index Array(array=w341, index (row)=1) -> (element=w338:string[])  [unwired: 1 in]
            n197 = Array Size(array=w338) -> (size(s)=w339:i32)
            n198 = for {
              N: w339 -> [_]
              tunnel: w338 -> [w347] mode=indexing
              i -> [w348]
              n199 = case shown="16" w348 {
                tunnel: w347 -> [w351 w354 w357 w360 w363 w366 w369 w372 w375 w377 w379 w381 w383 w385 w387 w389 w391 w393]
                frame 0, Default {
                  n200 = Fract/Exp String To Number(string=w351) -> (number=w350:dbl)  [unwired: 3 in, 1 out]
                  n201 = To Long Integer(number=w350) -> (32bit integer=w349:i32)
                  n202 = property on="Left LC1 zero point" class="DigNum (strict)"("Value"=w349) -> ()  [unwired: 2 in, 2 out]
                }
                frame 2 {
                  n203 = Fract/Exp String To Number(string=w354) -> (number=w353:dbl)  [unwired: 3 in, 1 out]
                  n204 = To Long Integer(number=w353) -> (32bit integer=w352:i32)
                  n205 = property on="Left LC2 zero point" class="DigNum (strict)"("Value"=w352) -> ()  [unwired: 2 in, 2 out]
                }
                frame 4 {
                  n206 = Fract/Exp String To Number(string=w357) -> (number=w356:dbl)  [unwired: 3 in, 1 out]
                  n207 = To Long Integer(number=w356) -> (32bit integer=w355:i32)
                  n208 = property on="Left LC3 zero point" class="DigNum (strict)"("Value"=w355) -> ()  [unwired: 2 in, 2 out]
                }
                frame 6 {
                  n209 = Fract/Exp String To Number(string=w360) -> (number=w359:dbl)  [unwired: 3 in, 1 out]
                  n210 = To Long Integer(number=w359) -> (32bit integer=w358:i32)
                  n211 = property on="Centre LC1 zero point" class="DigNum (strict)"("Value"=w358) -> ()  [unwired: 2 in, 2 out]
                }
                frame 8 {
                  n212 = Fract/Exp String To Number(string=w363) -> (number=w362:dbl)  [unwired: 3 in, 1 out]
                  n213 = To Long Integer(number=w362) -> (32bit integer=w361:i32)
                  n214 = property on="Centre LC2 zero point" class="DigNum (strict)"("Value"=w361) -> ()  [unwired: 2 in, 2 out]
                }
                frame 10 {
                  n215 = Fract/Exp String To Number(string=w366) -> (number=w365:dbl)  [unwired: 3 in, 1 out]
                  n216 = To Long Integer(number=w365) -> (32bit integer=w364:i32)
                  n217 = property on="Centre LC3 zero point" class="DigNum (strict)"("Value"=w364) -> ()  [unwired: 2 in, 2 out]
                }
                frame 12 {
                  n218 = Fract/Exp String To Number(string=w369) -> (number=w368:dbl)  [unwired: 3 in, 1 out]
                  n219 = To Long Integer(number=w368) -> (32bit integer=w367:i32)
                  n220 = property on="Right LC1 zero point" class="DigNum (strict)"("Value"=w367) -> ()  [unwired: 2 in, 2 out]
                }
                frame 14 {
                  n221 = Fract/Exp String To Number(string=w372) -> (number=w371:dbl)  [unwired: 3 in, 1 out]
                  n222 = To Long Integer(number=w371) -> (32bit integer=w370:i32)
                  n223 = property on="Right LC2 zero point" class="DigNum (strict)"("Value"=w370) -> ()  [unwired: 2 in, 2 out]
                }
                frame 16 {
                  n224 = Fract/Exp String To Number(string=w375) -> (number=w374:dbl)  [unwired: 3 in, 1 out]
                  n225 = To Long Integer(number=w374) -> (32bit integer=w373:i32)
                  n226 = property on="Right LC3 zero point" class="DigNum (strict)"("Value"=w373) -> ()  [unwired: 2 in, 2 out]
                }
                frame 1 {
                  n227 = Fract/Exp String To Number(string=w377) -> (number=w376:dbl)  [unwired: 3 in, 1 out]
                  n228 = property on="Left LC1 Calibration Constant" class="DigNum (strict)"("Value"=w376) -> ()  [unwired: 2 in, 2 out]
                }
                frame 3 {
                  n229 = Fract/Exp String To Number(string=w379) -> (number=w378:dbl)  [unwired: 3 in, 1 out]
                  n230 = property on="Left LC2 Calibration Constant" class="DigNum (strict)"("Value"=w378) -> ()  [unwired: 2 in, 2 out]
                }
                frame 5 {
                  n231 = Fract/Exp String To Number(string=w381) -> (number=w380:dbl)  [unwired: 3 in, 1 out]
                  n232 = property on="Left LC3 Calibration Constant" class="DigNum (strict)"("Value"=w380) -> ()  [unwired: 2 in, 2 out]
                }
                frame 7 {
                  n233 = Fract/Exp String To Number(string=w383) -> (number=w382:dbl)  [unwired: 3 in, 1 out]
                  n234 = property on="Centre LC1 Calibration Constant" class="DigNum (strict)"("Value"=w382) -> ()  [unwired: 2 in, 2 out]
                }
                frame 9 {
                  n235 = Fract/Exp String To Number(string=w385) -> (number=w384:dbl)  [unwired: 3 in, 1 out]
                  n236 = property on="Centre LC2 Calibration Constant" class="DigNum (strict)"("Value"=w384) -> ()  [unwired: 2 in, 2 out]
                }
                frame 11 {
                  n237 = Fract/Exp String To Number(string=w387) -> (number=w386:dbl)  [unwired: 3 in, 1 out]
                  n238 = property on="Centre LC3 Calibration Constant" class="DigNum (strict)"("Value"=w386) -> ()  [unwired: 2 in, 2 out]
                }
                frame 13 {
                  n239 = Fract/Exp String To Number(string=w389) -> (number=w388:dbl)  [unwired: 3 in, 1 out]
                  n240 = property on="Right LC1 Calibration Constant" class="DigNum (strict)"("Value"=w388) -> ()  [unwired: 2 in, 2 out]
                }
                frame 15 {
                  n241 = Fract/Exp String To Number(string=w391) -> (number=w390:dbl)  [unwired: 3 in, 1 out]
                  n242 = property on="Right LC2 Calibration Constant" class="DigNum (strict)"("Value"=w390) -> ()  [unwired: 2 in, 2 out]
                }
                frame 17 {
                  n243 = Fract/Exp String To Number(string=w393) -> (number=w392:dbl)  [unwired: 3 in, 1 out]
                  n244 = property on="Right LC3 Calibration Constant" class="DigNum (strict)"("Value"=w392) -> ()  [unwired: 2 in, 2 out]
                }
              }
            }
          }
        }
      }
    }
    n245 = Wait (ms)(milliseconds to wait=u32 50) -> ()  [unwired: 1 out]
  }
  n246 = xnode "Invoke Method"("FPGA VI Reference In"=w21) -> ("FPGA VI Reference Out"=w22:refnum<k20>)  [unwired: 1 in, 1 out]
  n247 = xnode "Close FPGA VI Reference"("FPGA VI Reference In"=w22) -> ()  [unwired: 1 in, 1 out]
  n248 = stacked-sequence {
    tunnel: [_ w405] -> w28
    tunnel: [_ w400] -> w27
    tunnel: [_ w399] -> w26
    tunnel: [_ w396] -> w24
    tunnel: w13 -> [_ _]
    frame #0 {
      n249 = Wait (ms)(milliseconds to wait=u32 100) -> ()  [unwired: 1 out]
    }
    frame #1 {
      n250 = xnode "Open FPGA VI Reference"() -> ("FPGA VI Reference Out"=w395:refnum<k20>)  [unwired: 2 in, 1 out]
      n251 = xnode "Invoke Method"("FPGA VI Reference In"=w395) -> ("FPGA VI Reference Out"=w396:refnum<k20>)  [unwired: 2 in, 1 out]
      n252 = Initialize Array(0.0 ("element"), 10 ("dimension size")) -> (w405:dbl[])
      n253 = Initialize Array(0.0 ("element"), 10 ("dimension size")) -> (w399:dbl[])
      n254 = Initialize Array(0.0 ("element"), 10 ("dimension size")) -> (w400:dbl[])
    }
  }
  n255 = while {
    tunnel: w24 -> [w415]
    tunnel: [w414] -> w25
    shift-right: [w411] -> _
    shift-left: w26 -> [w412]
    shift-right: [w408] -> _
    shift-left: w27 -> [w409]
    shift-right: [w407] -> _
    shift-left: w28 -> [w406]
    stop <- w416 stop-if-true
    # "Centre Stand"
    n256 = case shown="\"Main\", Default" "Centre Stand" {
      tunnel: w415 -> [w465 w505]
      tunnel: [w435 w500] -> w414
      tunnel: w412 -> [w457 w496]
      tunnel: [w421 w494] -> w411
      tunnel: w409 -> [w447 w486]
      tunnel: [w423 w484] -> w408
      tunnel: w406 -> [w437 w482]
      tunnel: [w422 w483] -> w407
      frame "Main", Default {
        n257 = xnode "Read/Write Control"("FPGA VI Reference In"=w465) -> ("FPGA VI Reference Out"=w464:refnum<k20>)  [unwired: 1 in, 2 out]
        n258 = Delete From Array(array=w447, length=1, index=0) -> (array with subset deleted=w448:dbl[])  [unwired: 1 out]
        n259 = Delete From Array(array=w437, length=1, index=0) -> (array with subset deleted=w441:dbl[])  [unwired: 1 out]
        n260 = Delete From Array(array=w457, length=1, index=0) -> (array with subset deleted=w460:dbl[])  [unwired: 1 out]
        n261 = xnode "Read/Write Control"("FPGA VI Reference In"=w464) -> ("FPGA VI Reference Out"=w463:refnum<k20>)  [unwired: 1 in, 2 out]
        n262 = xnode "Read/Write Control"("FPGA VI Reference In"=w463) -> ("FPGA VI Reference Out"=w462:refnum<k20>, "Data"=w453:i32)  [unwired: 1 in, 1 out]
        n263 = Build Array (concatenate)(w460, w453) -> (w421:dbl[])
        n264 = call-poly <vilib>:"Mean.vi"("X"=w421) -> ("mean"=w420:dbl)  [unwired: 1 out]
        n265 = property on="Centre LC1 zero point" class="DigNum (strict)"() -> ("Value"=w454:i32)  [unwired: 2 in, 2 out]
        n266 = property on="Centre LC2 zero point" class="DigNum (strict)"() -> ("Value"=w445:i32)  [unwired: 2 in, 2 out]
        n267 = Subtract(x=w420, y=w454) -> (x-y=w455:dbl)
        n268 = property on="Centre LC1 Calibration Constant" class="DigNum (strict)"() -> ("Value"=w456:dbl)  [unwired: 2 in, 2 out]
        n269 = property on="Centre LC3 zero point" class="DigNum (strict)"() -> ("Value"=w443:i32)  [unwired: 2 in, 2 out]
        n270 = property on="Centre LC2 Calibration Constant" class="DigNum (strict)"() -> ("Value"=w446:dbl)  [unwired: 2 in, 2 out]
        n271 = xnode "Read/Write Control"("FPGA VI Reference In"=w462) -> ("FPGA VI Reference Out"=w461:refnum<k20>, "Data 2"=w444:i32)  [unwired: 1 in, 1 out]
        n272 = Build Array (concatenate)(w448, w444) -> (w423:dbl[])
        n273 = call-poly <vilib>:"Mean.vi"("X"=w423) -> ("mean"=w418:dbl)  [unwired: 1 out]
        n274 = Subtract(x=w418, y=w445) -> (x-y=w451:dbl)
        n275 = property on="Centre LC3 Calibration Constant" class="DigNum (strict)"() -> ("Value"=w442:dbl)  [unwired: 2 in, 2 out]
        n276 = Multiply(x=w456, y=w455) -> (x*y=→"Centre Thrust":dbl)
        n277 = Multiply(x=w446, y=w451) -> (x*y=w425:dbl)
        "Centre LC2" <- w425
        n278 = xnode "Read/Write Control"("FPGA VI Reference In"=w461) -> ("FPGA VI Reference Out"=w435:refnum<k20>, "Data 3"=w436:i32)  [unwired: 1 in, 1 out]
        n279 = Build Array (concatenate)(w441, w436) -> (w422:dbl[])
        n280 = call-poly <vilib>:"Mean.vi"("X"=w422) -> ("mean"=w417:dbl)  [unwired: 1 out]
        n281 = Subtract(x=w417, y=w443) -> (x-y=w438:dbl)
        n282 = Multiply(x=w442, y=w438) -> (x*y=w426:dbl)
        "Centre LC3" <- w426
        n283 = local read "Tare All"() -> (w419:bool)
        n284 = Add(x=w425, y=w426) -> (x+y=w433:dbl)
        n285 = property on="Centre LC distance" class="DigNum (strict)"() -> ("Value"=w427:dbl)  [unwired: 2 in, 2 out]
        n286 = case shown="True" w419 {
          tunnel: w420 -> [_ w470]
          tunnel: [_ w469] -> _
          frame False {
          }
          frame True {
            n287 = property on="Centre LC1 zero point" class="DigNum (strict)"("Val(Sgnl)"=w470) -> (error out=w469:errorcluster)  [unwired: 2 in, 1 out]
          }
        }
        n288 = Divide(x=w427, y=2) -> (x/y=w432:dbl)
        n289 = case shown="True" w419 {
          tunnel: [_ w468] -> _
          tunnel: w418 -> [_ w467]
          tunnel: w417 -> [_ w466]
          frame False {
          }
          frame True {
            n290 = property on="Centre LC3 zero point" class="DigNum (strict)"("Val(Sgnl)"=w466) -> ()  [unwired: 2 in, 2 out]
            n291 = property on="Centre LC2 zero point" class="DigNum (strict)"("Val(Sgnl)"=w467) -> (error out=w468:errorcluster)  [unwired: 2 in, 1 out]
          }
        }
        n292 = Multiply(x=w432, y=w433) -> (x*y=w431:dbl)
        n293 = Divide(x=9.81, y=1000) -> (x/y=w428:dbl)
        n294 = Multiply(x=w431, y=w428) -> (x*y=→"Centre Torque":dbl)
      }
      frame "Setup" {
        n295 = xnode "Read/Write Control"("FPGA VI Reference In"=w505) -> ("FPGA VI Reference Out"=w504:refnum<k20>)  [unwired: 1 in, 2 out]
        n296 = Delete From Array(array=w496, length=1, index=0) -> (array with subset deleted=w495:dbl[])  [unwired: 1 out]
        n297 = Delete From Array(array=w482, length=1, index=0) -> (array with subset deleted=w479:dbl[])  [unwired: 1 out]
        n298 = Delete From Array(array=w486, length=1, index=0) -> (array with subset deleted=w489:dbl[])  [unwired: 1 out]
        n299 = xnode "Read/Write Control"("FPGA VI Reference In"=w504) -> ("FPGA VI Reference Out"=w503:refnum<k20>)  [unwired: 1 in, 2 out]
        n300 = xnode "Read/Write Control"("FPGA VI Reference In"=w503) -> ("FPGA VI Reference Out"=w502:refnum<k20>, "Data"=w492:i32)  [unwired: 1 in, 1 out]
        "Centre LC1 Reading" <- w492
        n301 = Build Array (concatenate)(w495, w492) -> (w494:dbl[])
        n302 = call-poly <vilib>:"Mean.vi"("X"=w494) -> ("mean"=w493:dbl)  [unwired: 1 out]
        n303 = xnode "Read/Write Control"("FPGA VI Reference In"=w502) -> ("FPGA VI Reference Out"=w501:refnum<k20>, "Data 2"=w485:i32)  [unwired: 1 in, 1 out]
        "Centre LC2 Reading" <- w485
        n304 = Build Array (concatenate)(w489, w485) -> (w484:dbl[])
        n305 = call-poly <vilib>:"Mean.vi"("X"=w484) -> ("mean"=w476:dbl)  [unwired: 1 out]
        n306 = case shown="True" "Centre LC1 Tare" {
          tunnel: w493 -> [_ w562]
          tunnel: [FALSE TRUE] -> _
          tunnel: [_ w560] -> _
          frame False {
          }
          frame True {
            n307 = property on="Centre LC1 zero point" class="DigNum (strict)"("Val(Sgnl)"=w562) -> (error out=w560:errorcluster)  [unwired: 2 in, 1 out]
          }
        }
        n308 = case shown="True" "Centre LC1 Calibrate" {
          tunnel: w493 -> [_ w558]
          frame False {
          }
          frame True {
            n309 = local read "Centre LC1 zero point"() -> (w557:i32)
            n310 = Subtract(x=w558, y=w557) -> (x-y=w556:dbl)
            n311 = Divide(x="Centre LC1 Calibration Weight (g)", y=w556) -> (x/y=→"Centre LC1 Calibration Constant":dbl)
          }
        }
        n312 = xnode "Read/Write Control"("FPGA VI Reference In"=w501) -> ("FPGA VI Reference Out"=w500:refnum<k20>, "Data 3"=w478:i32)  [unwired: 1 in, 1 out]
        "Centre LC3 Reading" <- w478
        n313 = Build Array (concatenate)(w479, w478) -> (w483:dbl[])
        n314 = call-poly <vilib>:"Mean.vi"("X"=w483) -> ("mean"=w477:dbl)  [unwired: 1 out]
        n315 = case shown="True" "Centre LC2 and LC3 measure 2" {
          tunnel: w477 -> [_ w540]
          tunnel: w476 -> [_ w539]
          frame False {
          }
          frame True {
            n316 = local read "Centre LC3 zero point"() -> (w542:i32)
            n317 = local read "Centre LC2 zero point"() -> (w541:i32)
            n318 = Subtract(x=w540, y=w542) -> (x-y=→"Centre LC3 Calibration measurement 2":dbl)
            n319 = Subtract(x=w539, y=w541) -> (x-y=→"Centre LC2 Calibration measurement 2":dbl)
          }
        }
        n320 = case shown="True" "Centre  LC2 and LC3 measure 1" {
          tunnel: w477 -> [_ w546]
          tunnel: w476 -> [_ w545]
          frame False {
          }
          frame True {
            n321 = local read "Centre LC2 zero point"() -> (w548:i32)
            n322 = local read "Centre LC3 zero point"() -> (w547:i32)
            n323 = Subtract(x=w545, y=w548) -> (x-y=→"Centre LC2 Calibration measurement 1":dbl)
            n324 = Subtract(x=w546, y=w547) -> (x-y=→"Centre LC3 Calibration measurement 1":dbl)
          }
        }
        n325 = case shown="True" "Centre LC3 Tare" {
          tunnel: w476 -> [_ w553]
          tunnel: [FALSE TRUE] -> _
          tunnel: [_ w551] -> _
          tunnel: w477 -> [_ w550]
          frame False {
          }
          frame True {
            n326 = property on="Centre LC3 zero point" class="DigNum (strict)"("Val(Sgnl)"=w550) -> ()  [unwired: 2 in, 2 out]
            n327 = property on="Centre LC2 zero point" class="DigNum (strict)"("Val(Sgnl)"=w553) -> (error out=w551:errorcluster)  [unwired: 2 in, 1 out]
          }
        }
        n328 = case shown="True" "Calibrate Torque" {
          frame False {
          }
          frame True {
            n329 = local read "Centre LC3 Calibration measurement 1"() -> (w515:dbl)
            n330 = local read "Centre LC3 Calibration measurement 2"() -> (w514:dbl)
            n331 = local read "Centre LC2 Calibration measurement 2"() -> (w513:dbl)
            n332 = local read "Centre LC2 Calibration measurement 1"() -> (w512:dbl)
            n333 = local read "Centre LC distance"() -> (w506:dbl)
            n334 = Multiply(x="Centre Calibration Weight 2 (g)", y=2) -> (x*y=w527:dbl)
            n335 = Multiply(x="Centre Calibration Weight 1 (g)", y=2) -> (x*y=w531:dbl)
            n336 = Multiply(x=w527, y="Centre Calibration arm 2 (m)") -> (x*y=w526:dbl)
            n337 = Multiply(x=w531, y="Centre Calibration arm 1 (m)") -> (x*y=w530:dbl)
            n338 = Divide(x=w526, y=w506) -> (x/y=w525:dbl)
            n339 = Divide(x=w530, y="Centre LC distance") -> (x/y=w529:dbl)
            n340 = Divide(x=w515, y=w514) -> (x/y=w524:dbl)
            n341 = Multiply(x=w524, y=w525) -> (x*y=w523:dbl)
            n342 = Subtract(x=w529, y=w523) -> (x-y=w522:dbl)
            n343 = Multiply(x=w524, y=w513) -> (x*y=w536:dbl)
            n344 = Divide(x=1, y=w514) -> (x/y=w520:dbl)
            n345 = Subtract(x=w512, y=w536) -> (x-y=w534:dbl)
            n346 = Divide(x=1, y=w534) -> (x/y=w533:dbl)
            n347 = Multiply(x=w533, y=w522) -> (x*y=w517:dbl)
            "Centre LC2 Calibration Constant" <- w517
            n348 = Multiply(x=w513, y=w517) -> (x*y=w518:dbl)
            n349 = Subtract(x=w525, y=w518) -> (x-y=w519:dbl)
            n350 = Multiply(x=w519, y=w520) -> (x*y=→"Centre LC3 Calibration Constant":dbl)
          }
        }
        n351 = Bundle(cluster=cluster{"Data":i32, "Data 2":i32, "Data 3":i32} {"Data"=0, "Data 2"=0, "Data 3"=0}, "Data"=w492, "Data 2"=w485, "Data 3"=w478) -> (→"Centre Raw Load Cell Readings":cluster{"Data":i32, "Data 2":i32, "Data 3":i32})
      }
    }
    n352 = Wait (ms)(milliseconds to wait=u32 5) -> ()  [unwired: 1 out]
    n353 = local read "StopLoops"() -> (w416:bool)
  }
  n354 = flat-sequence {
    frame #0 {
      # "Operating Mode"
      # "Torque Enable"
      # "Operating Mode"
      # "Torque Enable"
      n355 = flat-sequence {
        tunnel: [w674] -> w601
        tunnel: [w677] -> w566
        tunnel: w601 -> [w677]
        tunnel: [w676] -> _
        frame #0 {
          n356 = call <userlib>:"port Handler.vi"("port_name"="COM3") -> ("function return"=w674:i32)  [unwired: 9 in, 1 out]
          "function return" <- w674
        }
        frame #1 {
          n357 = call <userlib>:"packet Handler.vi"() -> ("error out"=w676:errorcluster)  [unwired: 11 in]
        }
      }
      n358 = flat-sequence {
        tunnel: w566 -> [w673]
        tunnel: [w671] -> w565
        frame #0 {
          n359 = call <userlib>:"open Port.vi"("port_num"=w673) -> ("error out"=w672:errorcluster)  [unwired: 9 in, 1 out]
          n360 = call <userlib>:"set Baud Rate.vi"("error in (no error)"=w672, "baudrate"=57600, "port_num"=w673) -> ("error out"=w671:errorcluster)  [unwired: 7 in, 1 out]
        }
      }
      n361 = call <userlib>:"write1Byte Tx Rx.vi"("data"=u32 1, "address"=u16 64, "error in (no error)"=w565, "id"=u8 1, "protocol_version"=2, "port_num"=w566) -> ("error out"=w581:errorcluster)  [unwired: 5 in]
      n362 = call <userlib>:"write1Byte Tx Rx.vi"("data"=u32 1, "address"=u16 64, "error in (no error)"=w581, "id"=u8 2, "protocol_version"=2, "port_num"=w566) -> ("error out"=w580:errorcluster)  [unwired: 5 in]
      n363 = call <userlib>:"write4Byte Tx Rx.vi"("data"="Motor 1 Operating Mode", "address"=u16 11, "error in (no error)"=w580, "id"=u8 1, "protocol_version"=2, "port_num"=w566) -> ("error out"=w575:errorcluster)  [unwired: 5 in]
      n364 = invoke on="Target Motor 1 Position" class="Slide (strict)" method="Reinit To Default"() -> (error out=w564:errorcluster)  [unwired: 3 in, 2 out]
      n365 = call <userlib>:"write4Byte Tx Rx.vi"("data"="Motor 2 Operating Mode", "address"=u16 11, "error in (no error)"=w575, "id"=u8 2, "protocol_version"=2, "port_num"=w566) -> ("error out"=w574:errorcluster)  [unwired: 5 in]
      n366 = invoke on="Target Motor 2 Position" class="Slide (strict)" method="Reinit To Default"() -> (error out=w563:errorcluster)  [unwired: 3 in, 2 out]
      n367 = while {
        tunnel: w566 -> [w635]
        shift-right: [w620] -> w588
        shift-left: w574 -> [w649]
        shift-right: [w643] -> _
        shift-left: u32 0 ("milliseconds to wait") -> [w645]
        tunnel: [w608] -> w569
        shift-right: [w624] -> _
        shift-left: u32 0 ("milliseconds to wait") -> [w626]
        tunnel: w564 -> [_]
        tunnel: w563 -> [_]
        stop <- w636 stop-if-true
        # "Motor 1"
        # "Motor 2"
        # "Get Position"
        # "Motor 2"
        # "Motor 1"
        # "Get Position"
        # "0-4095 = 0-360"
        # "Dynamixel Motors"
        n368 = local read "Dxl 1 Target Pos"() -> (w615:dbl)
        n369 = local read "Dxl 2 Target Pos"() -> (w614:dbl)
        n370 = Divide(x=4096.0 ("y"), y=360.0 ("x")) -> (x/y=w639:dbl)
        n371 = Multiply(x=w615, y=w639) -> (x*y=w646:dbl)
        n372 = To Word Integer(number=w646) -> (16bit integer=w642:i16)
        n373 = Not Equal?(x=w645, y=w642) -> (x != y?=w644:bool)
        n374 = Divide(x=4096.0 ("y"), y=360.0 ("x")) -> (x/y=w634:dbl)
        n375 = Multiply(x=w614, y=w634) -> (x*y=w631:dbl)
        n376 = Wait (ms)(milliseconds to wait=u32 10) -> ()  [unwired: 1 out]
        n377 = case shown="True" w644 {
          tunnel: w649 -> [w662 w666]
          tunnel: [w662 w665] -> w628
          tunnel: w635 -> [w660 w663]
          tunnel: w645 -> [w661 _]
          tunnel: [w661 w664] -> w643
          tunnel: w642 -> [_ w664]
          tunnel: [w660 w663] -> w629
          frame False {
          }
          frame True {
            # "Set Position"
            n378 = call <userlib>:"write4Byte Tx Rx.vi"("data"=w664, "address"=u16 116, "error in (no error)"=w666, "id"=u8 1, "protocol_version"=2, "port_num"=w663) -> ("error out"=w665:errorcluster)  [unwired: 5 in]
          }
        }
        n379 = To Word Integer(number=w631) -> (16bit integer=w625:i16)
        n380 = Not Equal?(x=w626, y=w625) -> (x != y?=w630:bool)
        n381 = case shown="True" w630 {
          tunnel: w628 -> [w652 w653]
          tunnel: [w652 w656] -> w627
          tunnel: w626 -> [w651 _]
          tunnel: [w651 w655] -> w624
          tunnel: w625 -> [_ w655]
          tunnel: [w650 w654] -> w608
          tunnel: w629 -> [w650 w654]
          frame False {
          }
          frame True {
            # "Set Position"
            n382 = call <userlib>:"write4Byte Tx Rx.vi"("data"=w655, "address"=u16 116, "error in (no error)"=w653, "id"=u8 2, "protocol_version"=2, "port_num"=w654) -> ("error out"=w656:errorcluster)  [unwired: 5 in]
          }
        }
        n383 = call <userlib>:"read4Byte Tx Rx.vi"("address"=u16 132, "error in (no error)"=w627, "id"=u8 1, "protocol_version"=2, "port_num"=w608) -> ("error out"=w606:errorcluster, "function return"=w605:u32)  [unwired: 5 in]
        n384 = Divide(x=4096.0, y=360.0) -> (x/y=w647:dbl)
        n385 = To Long Integer(number=w605) -> (32bit integer=w604:i32)
        "Position Raw 1" <- w604
        n386 = To Double Precision Float(number=w604) -> (double precision float=w613:dbl)
        n387 = Divide(x=w613, y=w647) -> (x/y=→"Current Motor 1 Position" →"Dxl 1 Pos":dbl)
        n388 = call <userlib>:"read4Byte Tx Rx.vi"("address"=u16 132, "error in (no error)"=w606, "id"=u8 2, "protocol_version"=2, "port_num"=w608) -> ("error out"=w620:errorcluster, "function return"=w602:u32)  [unwired: 5 in]
        n389 = To Long Integer(number=w602) -> (32bit integer=w603:i32)
        "Position Raw 2" <- w603
        n390 = Divide(x=4096.0, y=360.0) -> (x/y=w617:dbl)
        n391 = To Double Precision Float(number=w603) -> (double precision float=w612:dbl)
        n392 = Divide(x=w612, y=w617) -> (x/y=→"Current Motor 2 Position" →"Dxl 2 Pos":dbl)
        n393 = local read "StopLoops"() -> (w636:bool)
      }
      n394 = call <userlib>:"write1Byte Tx Rx.vi"("data"=u32 1, "address"=u16 64, "error in (no error)"=w588, "id"=u8 1, "protocol_version"=2, "port_num"=w569) -> ("error out"=w567:errorcluster)  [unwired: 5 in]
      n395 = call <userlib>:"write1Byte Tx Rx.vi"("data"=u32 1, "address"=u16 64, "error in (no error)"=w567, "id"=u8 2, "protocol_version"=2, "port_num"=w569) -> ("error out"=w568:errorcluster)  [unwired: 5 in]
      n396 = call <userlib>:"close Port.vi"("error in (no error)"=w568, "port_num"=w569) -> ()  [unwired: 9 in, 1 out]
    }
  }
  n397 = invoke on="Row Left" class="DigNum (strict)" method="Reinit To Default"() -> (error out=w8:errorcluster)  [unwired: 3 in, 2 out]
  n398 = xnode "Invoke Method"("FPGA VI Reference In"=w25) -> ("FPGA VI Reference Out"=w29:refnum<k20>)  [unwired: 1 in, 1 out]
  n399 = xnode "Close FPGA VI Reference"("FPGA VI Reference In"=w29) -> ()  [unwired: 1 in, 1 out]
  n400 = stacked-sequence {
    tunnel: [_ w698] -> w39
    tunnel: [_ w695] -> w36
    tunnel: [_ w694] -> w35
    tunnel: [_ w691] -> w34
    tunnel: [_ w688] -> w33
    tunnel: [_ w687] -> w32
    tunnel: [_ w684] -> w31
    tunnel: [_ w679] -> w30
    tunnel: w13 -> [_ _]
    frame #0 {
      n401 = Wait (ms)(milliseconds to wait=u32 100) -> ()  [unwired: 1 out]
    }
    frame #1 {
      n402 = xnode "Open FPGA VI Reference"() -> ("FPGA VI Reference Out"=w699:refnum<k20>)  [unwired: 2 in, 1 out]
      n403 = invoke on="Right PWM Slide" class="Slide (strict)" method="Reinit To Default"() -> (error out=w691:errorcluster)  [unwired: 3 in, 2 out]
      n404 = xnode "Invoke Method"("FPGA VI Reference In"=w699) -> ("FPGA VI Reference Out"=w698:refnum<k20>)  [unwired: 2 in, 1 out]
      n405 = Initialize Array(0.0 ("element"), 10 ("dimension size")) -> (w694:dbl[])
      n406 = Initialize Array(0.0 ("element"), 10 ("dimension size")) -> (w688:dbl[])
      n407 = Initialize Array(0.0 ("element"), 10 ("dimension size")) -> (w687:dbl[])
      n408 = Initialize Array(0.0 ("element"), 10 ("dimension size")) -> (w679:dbl[])
      n409 = Initialize Array(0.0 ("element"), 10 ("dimension size")) -> (w695:dbl[])
      n410 = Initialize Array(0.0 ("element"), 10 ("dimension size")) -> (w684:dbl[])
    }
  }
  n411 = String To Path(string="Control Table Path") -> (path=w9:path)
  n412 = invoke on="table input switch" class="Bool (strict)" method="Reinit To Default"() -> (error out=w11:errorcluster)  [unwired: 3 in, 2 out]
  n413 = invoke on="Row Right" class="DigNum (strict)" method="Reinit To Default"() -> (error out=w12:errorcluster)  [unwired: 3 in, 2 out]
  n414 = while {
    tunnel: w39 -> [w715]
    tunnel: [w714] -> w37
    shift-right: [w711] -> _
    shift-left: w36 -> [w712]
    shift-right: [w708] -> _
    shift-left: w35 -> [w709]
    tunnel: w34 -> [_]
    shift-right: [w706] -> _
    shift-left: w33 -> [w707]
    shift-right: [w704] -> _
    shift-left: w32 -> [w705]
    shift-right: [w702] -> _
    shift-left: w31 -> [w703]
    shift-right: [w701] -> _
    shift-left: w30 -> [w700]
    stop <- w716 stop-if-true
    # "Right Stand"
    n415 = case shown="\"Main\", Default" "Right Stand" {
      tunnel: w715 -> [w813 w865]
      tunnel: [w766 w860] -> w714
      tunnel: w712 -> [w805 w857]
      tunnel: [w733 w855] -> w711
      tunnel: w709 -> [w790 w853]
      tunnel: [w789 w853] -> w708
      tunnel: w707 -> [w773 w852]
      tunnel: [w768 w852] -> w706
      tunnel: w705 -> [w761 w848]
      tunnel: [w760 w848] -> w704
      tunnel: w703 -> [w755 w844]
      tunnel: [w732 w842] -> w702
      tunnel: w700 -> [w745 w840]
      tunnel: [w731 w841] -> w701
      frame "Main", Default {
        n416 = xnode "Read/Write Control"("FPGA VI Reference In"=w813) -> ("FPGA VI Reference Out"=w812:refnum<k20>, "RawVoltage"=w788:i16)  [unwired: 1 in, 1 out]
        n417 = Delete From Array(array=w755, length=1, index=0) -> (array with subset deleted=w756:dbl[])  [unwired: 1 out]
        n418 = Delete From Array(array=w745, length=1, index=0) -> (array with subset deleted=w749:dbl[])  [unwired: 1 out]
        n419 = Delete From Array(array=w773, length=1, index=0) -> (array with subset deleted=w772:dbl[])  [unwired: 1 out]
        n420 = Delete From Array(array=w790, length=1, index=0) -> (array with subset deleted=w796:dbl[])  [unwired: 1 out]
        n421 = Delete From Array(array=w805, length=1, index=0) -> (array with subset deleted=w808:dbl[])  [unwired: 1 out]
        n422 = xnode "Read/Write Control"("FPGA VI Reference In"=w812) -> ("FPGA VI Reference Out"=w811:refnum<k20>, "RawCurrent"=w769:u16)  [unwired: 1 in, 1 out]
        n423 = Build Array (concatenate)(w772, w769) -> (w768:dbl[])
        n424 = Build Array (concatenate)(w796, w788) -> (w789:dbl[])
        n425 = call-poly <vilib>:"Mean.vi"("X"=w768) -> ("mean"=w767:dbl)  [unwired: 1 out]
        n426 = call-poly <vilib>:"Mean.vi"("X"=w789) -> ("mean"=w794:dbl)  [unwired: 1 out]
        n427 = Divide(x=i16 20, y=i16 4096) -> (x/y=w795:dbl)
        n428 = Multiply(x=w794, y=w795) -> (x*y=w792:dbl)
        n429 = xnode "Read/Write Control"("FPGA VI Reference In"=w811) -> ("FPGA VI Reference Out"=w810:refnum<k20>, "Data"=w801:i32)  [unwired: 1 in, 1 out]
        n430 = Build Array (concatenate)(w808, w801) -> (w733:dbl[])
        n431 = call-poly <vilib>:"Mean.vi"("X"=w733) -> ("mean"=w721:dbl)  [unwired: 1 out]
        n432 = property on="Right LC1 zero point" class="DigNum (strict)"() -> ("Value"=w802:i32)  [unwired: 2 in, 2 out]
        n433 = property on="Right LC2 zero point" class="DigNum (strict)"() -> ("Value"=w753:i32)  [unwired: 2 in, 2 out]
        n434 = Add(x="Right Resistance Vout (Ohms)", y="Right Resistance non-Vout (Ohms)") -> (x+y=w787:dbl)
        n435 = Subtract(x=w721, y=w802) -> (x-y=w803:dbl)
        n436 = property on="Right LC1 Calibration Constant" class="DigNum (strict)"() -> ("Value"=w804:dbl)  [unwired: 2 in, 2 out]
        n437 = property on="Right LC3 zero point" class="DigNum (strict)"() -> ("Value"=w751:i32)  [unwired: 2 in, 2 out]
        n438 = property on="Right LC2 Calibration Constant" class="DigNum (strict)"() -> ("Value"=w754:dbl)  [unwired: 2 in, 2 out]
        n439 = xnode "Read/Write Control"("FPGA VI Reference In"=w810) -> ("FPGA VI Reference Out"=w809:refnum<k20>, "Data 2"=w752:i32)  [unwired: 1 in, 1 out]
        n440 = Build Array (concatenate)(w756, w752) -> (w732:dbl[])
        n441 = call-poly <vilib>:"Mean.vi"("X"=w732) -> ("mean"=w720:dbl)  [unwired: 1 out]
        n442 = Subtract(x=w720, y=w753) -> (x-y=w759:dbl)
        n443 = property on="Right LC3 Calibration Constant" class="DigNum (strict)"() -> ("Value"=w750:dbl)  [unwired: 2 in, 2 out]
        n444 = Divide(x=w787, y="Right Resistance Vout (Ohms)") -> (x/y=w791:dbl)
        n445 = Multiply(x=w791, y=w792) -> (x*y=w730:dbl)
        "Right Voltage" <- w730
        n446 = Divide(x=i16 5, y=i16 4096) -> (x/y=w783:dbl)
        n447 = Multiply(x=w804, y=w803) -> (x*y=w724:dbl)
        "Right Thrust" <- w724
        n448 = Multiply(x=w754, y=w759) -> (x*y=w723:dbl)
        "Right LC2" <- w723
        n449 = Multiply(x=w767, y=w783) -> (x*y=w774:dbl)
        n450 = Divide(x=i16 90 ("y"), y=3.3 ("x")) -> (x/y=w782:dbl)
        n451 = xnode "Read/Write Control"("FPGA VI Reference In"=w809) -> ("FPGA VI Reference Out"=w781:refnum<k20>, "Data 3"=w744:i32)  [unwired: 1 in, 1 out]
        n452 = Build Array (concatenate)(w749, w744) -> (w731:dbl[])
        n453 = call-poly <vilib>:"Mean.vi"("X"=w731) -> ("mean"=w719:dbl)  [unwired: 1 out]
        n454 = Subtract(x=w719, y=w751) -> (x-y=w746:dbl)
        n455 = Multiply(x=w750, y=w746) -> (x*y=w742:dbl)
        "Right LC3" <- w742
        n456 = Build Array(w724, w723) -> ()  [unwired: 1 out]
        n457 = Multiply(x=w774, y=w782) -> (x*y=w729:dbl)
        "Right Current" <- w729
        n458 = local read "PWM Right"() -> (w722:dbl)
        n459 = local read "Tare All"() -> (w718:bool)
        n460 = property on="Right LC distance" class="DigNum (strict)"() -> ("Value"=w739:dbl)  [unwired: 2 in, 2 out]
        n461 = Add(x=w723, y=w742) -> (x+y=w741:dbl)
        n462 = xnode "Read/Write Control"("FPGA VI Reference In"=w781, "Pulse Width (us)"=w722) -> ("FPGA VI Reference Out"=w780:refnum<k20>)  [unwired: 1 in, 1 out]
        n463 = case shown="True" w718 {
          tunnel: w721 -> [_ w818]
          tunnel: [_ w817] -> _
          frame False {
          }
          frame True {
            n464 = property on="Right LC1 zero point" class="DigNum (strict)"("Val(Sgnl)"=w818) -> (error out=w817:errorcluster)  [unwired: 2 in, 1 out]
          }
        }
        n465 = Divide(x=w739, y=2) -> (x/y=w740:dbl)
        n466 = Bundle(cluster=cluster{dbl, dbl} {0.0, 0.0}, w730, w729) -> (→"Waveform Chart":cluster{dbl, dbl})
        n467 = Multiply(x=w740, y=w741) -> (x*y=w738:dbl)
        n468 = Divide(x=9.81, y=1000) -> (x/y=w734:dbl)
        n469 = xnode "Read/Write Control"("FPGA VI Reference In"=w780, "Frequency"="Right PWM frequency") -> ("FPGA VI Reference Out"=w778:refnum<k20>)  [unwired: 1 in, 1 out]
        n470 = Multiply(x=w738, y=w734) -> (x*y=→"Right Torque":dbl)
        n471 = case shown="True" w718 {
          tunnel: w720 -> [_ w816]
          tunnel: [_ w815] -> _
          tunnel: w719 -> [_ w814]
          frame False {
          }
          frame True {
            n472 = property on="Right LC3 zero point" class="DigNum (strict)"("Val(Sgnl)"=w814) -> ()  [unwired: 2 in, 2 out]
            n473 = property on="Right LC2 zero point" class="DigNum (strict)"("Val(Sgnl)"=w816) -> (error out=w815:errorcluster)  [unwired: 2 in, 1 out]
          }
        }
        n474 = xnode "Read/Write Control"("FPGA VI Reference In"=w778, "PWM Switch"="Right PWM Switch") -> ("FPGA VI Reference Out"=w777:refnum<k20>)  [unwired: 1 in, 1 out]
        n475 = xnode "Read/Write Control"("FPGA VI Reference In"=w777) -> ("FPGA VI Reference Out"=w766:refnum<k20>, "Rotor Speed (Hz)"=w727:sgl)  [unwired: 1 in, 2 out]
        n476 = case shown="True" "Right PWM Switch" {
          tunnel: [0.0 ("Motor Frequency") w821] -> w726
          tunnel: w727 -> [_ w820]
          frame False {
          }
          frame True {
            w827 = T3 1 items=["RPM", "Hz"] ("Right Motor Units")
            n477 = Equal?(x="Right Motor Units", y=w827) -> (x = y?=w826:bool)
            n478 = Select(t=1.0, s=w826, f=60.0) -> (s? t:f=w822:dbl)
            n479 = Multiply(x=w822, y=w820) -> (x*y=w821:dbl)
          }
        }
        n480 = Delete From Array(array=w761, length=1, index=0) -> (array with subset deleted=w762:dbl[])  [unwired: 1 out]
        n481 = Build Array (concatenate)(w762, w726) -> (w760:dbl[])
        n482 = call-poly <vilib>:"Mean.vi"("X"=w760) -> ("mean"=→"Right Motor Frequency":dbl)  [unwired: 1 out]
      }
      frame "Setup" {
        n483 = xnode "Read/Write Control"("FPGA VI Reference In"=w865) -> ("FPGA VI Reference Out"=w864:refnum<k20>)  [unwired: 1 in, 2 out]
        n484 = Delete From Array(array=w840, length=1, index=0) -> (array with subset deleted=w837:dbl[])  [unwired: 1 out]
        n485 = Delete From Array(array=w857, length=1, index=0) -> (array with subset deleted=w856:dbl[])  [unwired: 1 out]
        n486 = Delete From Array(array=w844, length=1, index=0) -> (array with subset deleted=w847:dbl[])  [unwired: 1 out]
        n487 = xnode "Read/Write Control"("FPGA VI Reference In"=w864) -> ("FPGA VI Reference Out"=w863:refnum<k20>)  [unwired: 1 in, 2 out]
        n488 = xnode "Read/Write Control"("FPGA VI Reference In"=w863) -> ("FPGA VI Reference Out"=w862:refnum<k20>, "Data"=w851:i32)  [unwired: 1 in, 1 out]
        "Right LC1 Reading" <- w851
        n489 = Build Array (concatenate)(w856, w851) -> (w855:dbl[])
        n490 = call-poly <vilib>:"Mean.vi"("X"=w855) -> ("mean"=w854:dbl)  [unwired: 1 out]
        n491 = xnode "Read/Write Control"("FPGA VI Reference In"=w862) -> ("FPGA VI Reference Out"=w861:refnum<k20>, "Data 2"=w843:i32)  [unwired: 1 in, 1 out]
        "Right LC2 Reading" <- w843
        n492 = Build Array (concatenate)(w847, w843) -> (w842:dbl[])
        n493 = call-poly <vilib>:"Mean.vi"("X"=w842) -> ("mean"=w834:dbl)  [unwired: 1 out]
        n494 = case shown="True" "Right LC1 Tare" {
          tunnel: w854 -> [_ w922]
          tunnel: [_ w921] -> _
          frame False {
          }
          frame True {
            n495 = property on="Right LC1 zero point" class="DigNum (strict)"("Val(Sgnl)"=w922) -> (error out=w921:errorcluster)  [unwired: 2 in, 1 out]
          }
        }
        n496 = case shown="True" "Right LC1 Calibrate" {
          tunnel: w854 -> [_ w920]
          frame False {
          }
          frame True {
            n497 = local read "Right LC1 zero point"() -> (w919:i32)
            n498 = Subtract(x=w920, y=w919) -> (x-y=w918:dbl)
            n499 = Divide(x="Right LC1 Calibration Weight (kg)", y=w918) -> (x/y=→"Right LC1 Calibration Constant":dbl)
          }
        }
        n500 = xnode "Read/Write Control"("FPGA VI Reference In"=w861) -> ("FPGA VI Reference Out"=w860:refnum<k20>, "Data 3"=w836:i32)  [unwired: 1 in, 1 out]
        "Right LC3 Reading" <- w836
        n501 = Build Array (concatenate)(w837, w836) -> (w841:dbl[])
        n502 = call-poly <vilib>:"Mean.vi"("X"=w841) -> ("mean"=w835:dbl)  [unwired: 1 out]
        n503 = case shown="True" "Right LC2 and LC3 measure 1" {
          tunnel: w834 -> [_ w910]
          tunnel: w835 -> [_ w907]
          tunnel: [FALSE TRUE] -> _
          frame False {
          }
          frame True {
            n504 = local read "Right LC2 zero point"() -> (w909:i32)
            n505 = local read "Right LC3 zero point"() -> (w908:i32)
            n506 = Subtract(x=w910, y=w909) -> (x-y=→"Right LC2 Calibration measurement 1":dbl)
            n507 = Subtract(x=w907, y=w908) -> (x-y=→"Right LC3 Calibration measurement 1":dbl)
          }
        }
        n508 = case shown="True" "Right LC2 and LC3 measure 2" {
          tunnel: w835 -> [_ w900]
          tunnel: w834 -> [_ w899]
          frame False {
          }
          frame True {
            n509 = local read "Right LC2 zero point"() -> (w902:i32)
            n510 = local read "Right LC3 zero point"() -> (w901:i32)
            n511 = Subtract(x=w900, y=w901) -> (x-y=→"Right LC3 Calibration measurement 2":dbl)
            n512 = Subtract(x=w899, y=w902) -> (x-y=→"Right LC2 Calibration measurement 2":dbl)
          }
        }
        n513 = case shown="True" "Right LC2 and LC3 Tare" {
          tunnel: w834 -> [_ w915]
          tunnel: [FALSE TRUE] -> _
          tunnel: [_ w913] -> _
          tunnel: w835 -> [_ w912]
          frame False {
          }
          frame True {
            n514 = property on="Right LC2 zero point" class="DigNum (strict)"("Val(Sgnl)"=w915) -> (error out=w913:errorcluster)  [unwired: 2 in, 1 out]
            n515 = property on="Right LC3 zero point" class="DigNum (strict)"("Val(Sgnl)"=w912) -> ()  [unwired: 2 in, 2 out]
          }
        }
        n516 = case shown="True" "Toque calibrate" {
          frame False {
          }
          frame True {
            n517 = local read "Right LC distance"() -> (w880:dbl)
            n518 = local read "Right LC3 Calibration measurement 2"() -> (w873:dbl)
            n519 = local read "Right LC2 Calibration measurement 2"() -> (w871:dbl)
            n520 = local read "Right LC2 Calibration measurement 1"() -> (w895:dbl)
            n521 = local read "Right LC3 Calibration measurement 1"() -> (w896:dbl)
            n522 = Multiply(x="Right Calibration Weight 2 (g)", y=2) -> (x*y=w883:dbl)
            n523 = Multiply(x="Right Calibration Weight 1 (g)", y=2) -> (x*y=w891:dbl)
            n524 = Multiply(x=w883, y="Right Calibration arm 2 (m)") -> (x*y=w885:dbl)
            n525 = Multiply(x=w891, y="Right Calibration arm 1 (m)") -> (x*y=w887:dbl)
            n526 = Divide(x=w885, y=w880) -> (x/y=w872:dbl)
            n527 = Divide(x=w887, y="Right LC distance") -> (x/y=w878:dbl)
            n528 = Divide(x=w896, y=w873) -> (x/y=w879:dbl)
            n529 = Multiply(x=w879, y=w872) -> (x*y=w877:dbl)
            n530 = Subtract(x=w878, y=w877) -> (x-y=w875:dbl)
            n531 = Multiply(x=w879, y=w871) -> (x*y=w894:dbl)
            n532 = Divide(x=1, y=w873) -> (x/y=w868:dbl)
            n533 = Subtract(x=w895, y=w894) -> (x-y=w892:dbl)
            n534 = Divide(x=1, y=w892) -> (x/y=w876:dbl)
            n535 = Multiply(x=w876, y=w875) -> (x*y=w870:dbl)
            "Right LC2 Calibration Constant" <- w870
            n536 = Multiply(x=w871, y=w870) -> (x*y=w869:dbl)
            n537 = Subtract(x=w872, y=w869) -> (x-y=w867:dbl)
            n538 = Multiply(x=w867, y=w868) -> (x*y=→"Right LC3 Calibration Constant":dbl)
          }
        }
        n539 = Bundle(cluster=cluster{"Data":i32, "Data 2":i32, "Data 3":i32} {"Data"=0, "Data 2"=0, "Data 3"=0}, "Data"=w851, "Data 2"=w843, "Data 3"=w836) -> (→"Right Raw Load Cell Readings":cluster{"Data":i32, "Data 2":i32, "Data 3":i32})
      }
    }
    n540 = Wait (ms)(milliseconds to wait=u32 5) -> ()  [unwired: 1 out]
    n541 = local read "StopLoops"() -> (w716:bool)
  }
  n542 = invoke on="Closed loop" class="Bool (strict)" method="Reinit To Default"() -> (error out=w5:errorcluster)  [unwired: 3 in, 2 out]
  n543 = invoke on="Row Dxl 1" class="DigNum (strict)" method="Reinit To Default"() -> (error out=w7:errorcluster)  [unwired: 3 in, 2 out]
  n544 = invoke on="Row Dxl 2" class="DigNum (strict)" method="Reinit To Default"() -> (error out=w6:errorcluster)  [unwired: 3 in, 2 out]
  n545 = flat-sequence {
    frame #0 {
      n546 = Format Date/Time String(time format string (%c)="%Y_%m_%d_%H_%M_%S") -> (date/time string=w933:string)  [unwired: 2 in]
      n547 = Concatenate Strings("Data  Save Path", "\\data" ("name or relative path")) -> (w932:string)
      n548 = invoke on="Counts" class="DigNum (strict)" method="Reinit To Default"() -> (error out=w923:errorcluster)  [unwired: 3 in, 2 out]
      n549 = Concatenate Strings(w932, w933) -> (w934:string)
      n550 = invoke on="StopLoops" class="Bool (strict)" method="Reinit To Default"() -> (error out=w924:errorcluster)  [unwired: 3 in, 2 out]
      n551 = Concatenate Strings(w934, ".csv" ("name or relative path")) -> (w935:string)
      n552 = String To Path(string=w935) -> (path=w936:path)
      n553 = call-poly <vilib>:"Write Delimited Spreadsheet.vi"("file path (dialog if empty)"=w936, "1D data"=string[] ["PWM Left", "PWM Right", "Dxl 1 Pos ", "Dxl 2 Pos ", "Thrust Left [g]", "Torque Left [Nm]", "Thrust Right [g]", "Torque Right [Nm]", "Thrust Centre [g]", "Torque Centre [Nm]", "Voltage Left [V]", "Voltage Right [V]", "Current Left [A]", "Current Right [A]", "Speed Left [rpm]", "Speed Right [rpm]", "Total Thrust [g]", "Total Torque [Nm]", "Time [s]"], "delimiter (\\t)"="," ("delimiter (\\t)")) -> ("new file path (Not A Path if cancelled)"=w926:path)  [unwired: 11 in, 1 out]
      n554 = while {
        tunnel: w926 -> [w938]
        tunnel: w924 -> [_]
        tunnel: w923 -> [_]
        stop <- w939 stop-if-true
        # "Recordings"
        n555 = Wait (ms)(milliseconds to wait=u32 1) -> ()  [unwired: 1 out]
        n556 = event shown="[0] \"Record data\": Value Change" {
          selector: _ -> [_]
          dyn-events: _ -> [_]
          timeout: _ -> [_]
          tunnel: w938 -> [w942]
          event "Record data": Value Change {
            n557 = event-data() -> ("Time"=w940:u32, "NewVal"=w941:bool)  [unwired: 1 in, 4 out]
            n558 = case shown="True" w941 {
              tunnel: w942 -> [_ w971]
              tunnel: w940 -> [_ w944]
              frame False {
              }
              frame True {
                n559 = local read "Current Motor 1 Position"() -> (w949:dbl)
                n560 = local read "Current Motor 2 Position"() -> (w948:dbl)
                n561 = local read "Right Motor Frequency"() -> (w962:dbl)
                n562 = local read "Left Motor Frequency"() -> (w953:dbl)
                n563 = local read "Left Torque"() -> (w956:dbl)
                n564 = local read "Left Thrust"() -> (w957:dbl)
                n565 = local read "Centre Torque"() -> (w950:dbl)
                n566 = local read "Total Thrust"() -> (w947:dbl)
                n567 = local read "Centre Thrust"() -> (w951:dbl)
                n568 = local read "Right Current"() -> (w963:dbl)
                n569 = local read "PWM Right"() -> (w967:dbl)
                n570 = local read "Right Torque"() -> (w965:dbl)
                n571 = local read "PWM Left"() -> (w958:dbl)
                n572 = local read "Right Voltage"() -> (w964:dbl)
                n573 = local read "Right Thrust"() -> (w966:dbl)
                n574 = local read "Left Voltage"() -> (w955:dbl)
                n575 = local read "Left Current"() -> (w954:dbl)
                n576 = local read "Total Torque"() -> (w946:dbl)
                n577 = local read "Counts"() -> (w960:i32)
                n578 = Multiply(x=w944, y=0.001) -> (x*y=w943:dbl)
                n579 = Build Array (concatenate)(dbl[] [], w958, w967, w949, w948, w957, w956, w966, w965, w951, w950, w955, w964, w954, w963, w953, w962, w947, w946, w943) -> (w968:dbl[])
                n580 = Increment(x=w960) -> (x+1=→"Counts":i32)
                n581 = call-poly <vilib>:"Write Delimited Spreadsheet.vi"("file path (dialog if empty)"=w971, "format (%.3f)"="%.8f", "1D data"=w968, "append to file? (new file:F)"=TRUE, "delimiter (\\t)"="," ("delimiter (\\t)")) -> ()  [unwired: 9 in, 2 out]
              }
            }
          }
        }
        n582 = local read "StopLoops"() -> (w939:bool)
      }
    }
  }
  n583 = invoke on="Thrust Row" class="DigNum (strict)" method="Reinit To Default"() -> (error out=w4:errorcluster)  [unwired: 3 in, 2 out]
  n584 = xnode "Invoke Method"("FPGA VI Reference In"=w37) -> ("FPGA VI Reference Out"=w38:refnum<k20>)  [unwired: 1 in, 1 out]
  n585 = xnode "Close FPGA VI Reference"("FPGA VI Reference In"=w38) -> ()  [unwired: 1 in, 1 out]
  n586 = invoke on="Torque Row" class="DigNum (strict)" method="Reinit To Default"() -> (error out=w3:errorcluster)  [unwired: 3 in, 2 out]
  n587 = invoke on="Total Desired Torque [Nm]" class="DigNum (strict)" method="Reinit To Default"() -> (error out=w2:errorcluster)  [unwired: 3 in, 2 out]
  n588 = invoke on="Total Desired Thrust [g]" class="DigNum (strict)" method="Reinit To Default"() -> (error out=w1:errorcluster)  [unwired: 3 in, 2 out]
  n589 = while {
    tunnel: w12 -> [_]
    tunnel: w11 -> [_]
    tunnel: w9 -> [w1023]
    tunnel: w8 -> [_]
    tunnel: w7 -> [_]
    tunnel: w6 -> [_]
    tunnel: w5 -> [_]
    tunnel: w4 -> [_]
    tunnel: w3 -> [_]
    tunnel: w2 -> [_]
    tunnel: w1 -> [_]
    stop <- w1016 stop-if-true
    # "Control"
    n590 = local read "Closed Loop Left output"() -> (w999:dbl)
    n591 = call-poly <vilib>:"Read Delimited Spreadsheet.vi"("file path (dialog if empty)"=w1023, "delimiter (\\t)"="," ("delimiter (\\t)")) -> ("all rows"=w979:string[][])  [unwired: 8 in, 5 out]
    "Table Control" <- w979
    n592 = Array Size(array=w979) -> (size(s)=w978:i32[])
    n593 = Index Array(array=w978, index=0) -> (element=w976:i32)
    n594 = Subtract(x=w976, y=1) -> (x-y=w975:i32)
    "# of Control Rows" <- w975
    n595 = case "Left Rotor Table Control" shown="True" "table input switch" {
      tunnel: [1000 w1269] -> w1019
      tunnel: "Row Left" -> [_ w1266]
      tunnel: w975 -> [_ w1265]
      tunnel: "Collum Left" -> [_ w1264]
      tunnel: w979 -> [_ w1263]
      tunnel: "Closed loop" -> [_ w1261]
      frame False {
      }
      frame True {
        n596 = Subtract(x=w1266, y=1) -> (x-y=w1273:dbl)
        n597 = Greater?(x=w1266, y=w1265) -> (0:w1268:bool)
        n598 = Index Array(array=w1263, index (row) #1=w1266, index (col) #1=w1264, index (row) #2=w1273, index (col) #2=w1264) -> (element #1=w1275:string, element #2=w1272:string)
        n599 = local read "Setlting time [s]"() -> (w1262:i32)
        n600 = local write "StopLoops"(w1268) -> ()
        n601 = Fract/Exp String To Number(string=w1272) -> (number=w1270:dbl)  [unwired: 3 in, 1 out]
        n602 = Fract/Exp String To Number(string=w1275) -> (number=w1271:dbl)  [unwired: 3 in, 1 out]
        n603 = flat-sequence {
          tunnel: w1271 -> [w1285]
          tunnel: w1270 -> [w1283]
          tunnel: [w1277] -> w1269
          tunnel: [w1276] -> w1259
          frame #0 {
            w1279 = 1
            n604 = call "Is Value Changed.vim"("value"=w1285) -> ("changed or first call?"=w1286:bool)
            n605 = Subtract(x=w1285, y=w1283) -> (x-y=w1284:dbl)
            n606 = call "Elapsed Time2"("Reset"=w1286) -> ("Elapsed Time (s)"=w1276:dbl)  [unwired: 11 in, 7 out]
            n607 = Divide(x=w1276, y=2) -> (x/y=w1278:dbl)
            n608 = Greater?(x=w1278, y=w1279) -> (0:w1280:bool)
            n609 = Select(t=w1279, s=w1280, f=w1278) -> (s? t:f=w1281:dbl)
            n610 = Multiply(x=w1281, y=w1284) -> (x*y=w1282:dbl)
            n611 = Add(x=w1282, y=w1283) -> (x+y=w1277:dbl)
          }
        }
        n612 = local read "Time under tolerance"() -> (w1258:dbl)
        n613 = Select(t=w1258, s=w1261, f=w1259) -> (s? t:f=w1260:dbl)
        n614 = Greater?(x=w1260, y=w1262) -> (0:w1267:bool)
        n615 = case shown="True" w1267 {
          tunnel: w1261 -> [_ w1288]
          frame False {
          }
          frame True {
            n616 = case shown="True" w1288 {
              frame False {
                n617 = local read "Row Left"() -> (w1289:dbl)
                n618 = Increment(x=w1289) -> (x+1=w1290:dbl)
                n619 = local write "Row Left"(w1290) -> ()
              }
              frame True {
                n620 = local read "Row Dxl 1"() -> (w1291:dbl)
                n621 = local write "Row Left"(w1291) -> ()
              }
            }
          }
        }
        "Timer Left" <- w1259
      }
    }
    n622 = Select(t=w1019, s="table input switch", f="Left PWM pulse width") -> (s? t:f=w1000:dbl)
    n623 = Select(t=w999, s="Closed loop", f=w1000) -> (s? t:f=→"PWM Left" →"PWM Left":dbl)
    n624 = case "Right Rotor Table Control" shown="True" "table input switch" {
      tunnel: [1000 w1295] -> w1024
      tunnel: "Row Right" -> [_ w1304]
      tunnel: w975 -> [_ w1303]
      tunnel: "Collum Right" -> [_ w1302]
      tunnel: w979 -> [_ w1301]
      tunnel: "Closed loop" -> [_ w1299]
      frame False {
      }
      frame True {
        n625 = Subtract(x=w1304, y=1) -> (x-y=w1308:dbl)
        n626 = Greater?(x=w1304, y=w1303) -> (0:w1305:bool)
        n627 = Index Array(array=w1301, index (row) #1=w1304, index (col) #1=w1302, index (row) #2=w1308, index (col) #2=w1302) -> (element #1=w1310:string, element #2=w1307:string)
        n628 = local write "StopLoops"(w1305) -> ()
        n629 = Fract/Exp String To Number(string=w1307) -> (number=w1293:dbl)  [unwired: 3 in, 1 out]
        n630 = Fract/Exp String To Number(string=w1310) -> (number=w1294:dbl)  [unwired: 3 in, 1 out]
        n631 = flat-sequence {
          tunnel: w1294 -> [w1320]
          tunnel: w1293 -> [w1318]
          tunnel: [w1312] -> w1295
          tunnel: [w1311] -> w1296
          frame #0 {
            w1314 = 1
            n632 = call "Is Value Changed.vim"("value"=w1320) -> ("changed or first call?"=w1321:bool)
            n633 = Subtract(x=w1320, y=w1318) -> (x-y=w1319:dbl)
            n634 = call "Elapsed Time"("Reset"=w1321) -> ("Elapsed Time (s)"=w1311:dbl)  [unwired: 11 in, 7 out]
            n635 = Divide(x=w1311, y=2) -> (x/y=w1313:dbl)
            n636 = Greater?(x=w1313, y=w1314) -> (0:w1315:bool)
            n637 = Select(t=w1314, s=w1315, f=w1313) -> (s? t:f=w1316:dbl)
            n638 = Multiply(x=w1316, y=w1319) -> (x*y=w1317:dbl)
            n639 = Add(x=w1317, y=w1318) -> (x+y=w1312:dbl)
          }
        }
        n640 = local read "Time under tolerance"() -> (w1297:dbl)
        n641 = Select(t=w1297, s=w1299, f=w1296) -> (s? t:f=w1298:dbl)
        n642 = Greater?(x=w1298, y="Setlting time [s]") -> (0:w1300:bool)
        n643 = case shown="True" w1300 {
          selector: w1300 -> [_ w1323]
          tunnel: w1299 -> [_ w1324]
          frame False {
          }
          frame True {
            n644 = case shown="True" w1324 {
              tunnel: w1323 -> [w1325 _]
              frame False {
                n645 = local read "Row Right"() -> (w1326:dbl)
                n646 = Increment(x=w1326) -> (x+1=w1327:dbl)
                n647 = local write "Row Right"(w1327) -> ()
                n648 = property on="Record data" class="Bool (strict)"("Val(Sgnl)"=w1325) -> ()  [unwired: 2 in, 2 out]
              }
              frame True {
                n649 = local read "Row Dxl 1"() -> (w1328:dbl)
                n650 = local write "Row Right"(w1328) -> ()
              }
            }
          }
        }
        "Timer Right" <- w1296
      }
    }
    n651 = Wait (ms)(milliseconds to wait=u32 5) -> ()  [unwired: 1 out]
    n652 = call "Is Value Changed.vim"("value"="table input switch") -> ("changed or first call?"=w982:bool)
    n653 = call "Is Value Changed.vim"("value"="Closed loop") -> ("changed or first call?"=w981:bool)
    n654 = Or(x=w981, y=w982) -> (x .or. y?=w980:bool)
    n655 = case shown="True" w980 {
      frame False {
      }
      frame True {
        n656 = local write "Time under tolerance"(0.0) -> ()
      }
    }
    n657 = local read "StopLoops"() -> (w1016:bool)
    n658 = local read "Closed Loop Right output"() -> (w1002:dbl)
    n659 = Select(t=w1024, s="table input switch", f="Right PWM Slide") -> (s? t:f=w1003:dbl)
    n660 = Select(t=w1002, s="Closed loop", f=w1003) -> (s? t:f=→"PWM Right" →"PWM Right":dbl)
    n661 = case "Dynamixel Table Control" shown="True" "table input switch" {
      tunnel: [0 w1234] -> w1012
      tunnel: "Row Dxl 1" -> [_ w1231]
      tunnel: w975 -> [_ w1230]
      tunnel: "Collum Dxl 1" -> [_ w1212]
      tunnel: w979 -> [_ w1213]
      tunnel: "Collum Dxl 2" -> [_ w1211]
      tunnel: "Row Dxl 2" -> [_ w1210]
      tunnel: w975 -> [_ w1209]
      tunnel: [0 w1208] -> w1005
      tunnel: "Closed loop" -> [_ w1200]
      frame False {
      }
      frame True {
        w1226 = 1
        w1236 = 1
        n662 = Greater?(x=w1231, y=w1230) -> (0:w1233:bool)
        n663 = local write "StopLoops"(w1233) -> ()
        n664 = Subtract(x=w1210, y=1) -> (x-y=w1216:dbl)
        n665 = Subtract(x=w1231, y=1) -> (x-y=w1246:dbl)
        n666 = Greater?(x=w1210, y=w1209) -> (0:w1228:bool)
        n667 = Index Array(array=w1213, index (row) #1=w1210, index (col) #1=w1211, index (row) #2=w1216, index (col) #2=w1211) -> (element #1=w1214:string, element #2=w1217:string)
        n668 = Index Array(array=w1213, index (row) #1=w1231, index (col) #1=w1212, index (row) #2=w1246, index (col) #2=w1212) -> (element #1=w1248:string, element #2=w1245:string)
        n669 = local write "StopLoops"(w1228) -> ()
        n670 = local read "Setlting time [s]"() -> (w1206:i32)
        n671 = local read "Setlting time [s]"() -> (w1207:i32)
        n672 = Fract/Exp String To Number(string=w1217) -> (number=w1222:dbl)  [unwired: 3 in, 1 out]
        n673 = Fract/Exp String To Number(string=w1214) -> (number=w1220:dbl)  [unwired: 3 in, 1 out]
        n674 = Fract/Exp String To Number(string=w1245) -> (number=w1240:dbl)  [unwired: 3 in, 1 out]
        n675 = Fract/Exp String To Number(string=w1248) -> (number=w1242:dbl)  [unwired: 3 in, 1 out]
        n676 = call "Is Value Changed.vim"("value"=w1220) -> ("changed or first call?"=w1219:bool)
        n677 = Subtract(x=w1220, y=w1222) -> (x-y=w1221:dbl)
        n678 = call "Is Value Changed.vim"("value"=w1242) -> ("changed or first call?"=w1243:bool)
        n679 = Subtract(x=w1242, y=w1240) -> (x-y=w1241:dbl)
        n680 = call "Elapsed Time4"("Reset"=w1219) -> ("Elapsed Time (s)"=w1204:dbl)  [unwired: 11 in, 7 out]
        "Timer Dxl 2" <- w1204
        n681 = call "Elapsed Time3"("Reset"=w1243) -> ("Elapsed Time (s)"=w1201:dbl)  [unwired: 11 in, 7 out]
        "Timer Dxl 1" <- w1201
        n682 = Divide(x=w1204, y=1) -> (x/y=w1227:dbl)
        n683 = Divide(x=w1201, y=1) -> (x/y=w1235:dbl)
        n684 = Greater?(x=w1227, y=w1226) -> (0:w1225:bool)
        n685 = Greater?(x=w1235, y=w1236) -> (0:w1237:bool)
        n686 = local read "Time under tolerance"() -> (w1199:dbl)
        n687 = Select(t=w1199, s=w1200, f=w1201) -> (s? t:f=w1202:dbl)
        n688 = Greater?(x=w1202, y=w1207) -> (0:w1232:bool)
        n689 = case shown="True" w1232 {
          selector: w1232 -> [_ w1251]
          tunnel: w1200 -> [_ w1252]
          frame False {
          }
          frame True {
            n690 = local read "Row Dxl 1"() -> (w1254:dbl)
            n691 = case shown="True" w1252 {
              tunnel: w1251 -> [_ w1256]
              frame False {
              }
              frame True {
                n692 = property on="Record data" class="Bool (strict)"("Val(Sgnl)"=w1256) -> ()  [unwired: 2 in, 2 out]
                n693 = local write "Time under tolerance"(0.0) -> ()
              }
            }
            n694 = Increment(x=w1254) -> (x+1=w1253:dbl)
            n695 = local write "Row Dxl 1"(w1253) -> ()
          }
        }
        n696 = local read "Time under tolerance"() -> (w1203:dbl)
        n697 = Select(t=w1203, s=w1200, f=w1204) -> (s? t:f=w1205:dbl)
        n698 = Greater?(x=w1205, y=w1206) -> (0:w1229:bool)
        n699 = case shown="True" w1229 {
          frame False {
          }
          frame True {
            n700 = local read "Row Dxl 2"() -> (w1250:dbl)
            n701 = Increment(x=w1250) -> (x+1=w1249:dbl)
            n702 = local write "Row Dxl 2"(w1249) -> ()
          }
        }
        n703 = Select(t=w1226, s=w1225, f=w1227) -> (s? t:f=w1224:dbl)
        n704 = Select(t=w1236, s=w1237, f=w1235) -> (s? t:f=w1238:dbl)
        n705 = Multiply(x=w1224, y=w1221) -> (x*y=w1223:dbl)
        n706 = Multiply(x=w1238, y=w1241) -> (x*y=w1239:dbl)
        n707 = Add(x=w1223, y=w1222) -> (x+y=w1208:dbl)
        n708 = Add(x=w1239, y=w1240) -> (x+y=w1234:dbl)
      }
    }
    n709 = local read "Centre Thrust"() -> (w996:dbl)
    n710 = local read "Right Thrust"() -> (w998:dbl)
    n711 = local read "Left Thrust"() -> (w997:dbl)
    n712 = local read "Row Dxl 1"() -> (w984:dbl)
    n713 = Select(t=w1005, s="table input switch", f="Target Motor 2 Position") -> (s? t:f=→"Dxl 2 Target Pos":dbl)
    n714 = Select(t=w1012, s="table input switch", f="Target Motor 1 Position") -> (s? t:f=→"Dxl 1 Target Pos":dbl)
    n715 = local write "Torque Row"(w984) -> ()
    n716 = Add(x=w996, y=w997) -> (x+y=w995:dbl)
    n717 = local write "Thrust Row"(w984) -> ()
    n718 = Add(x=w995, y=w998) -> (x+y=w994:dbl)
    "Total Thrust" <- w994
    n719 = local read "Centre Torque"() -> (w991:dbl)
    n720 = local read "Right Torque"() -> (w993:dbl)
    n721 = local read "Left Torque"() -> (w992:dbl)
    n722 = Add(x=w991, y=w992) -> (x+y=w990:dbl)
    n723 = Add(x=w990, y=w993) -> (x+y=w989:dbl)
    "Total Torque" <- w989
    n724 = call "Is Value Changed.vim"("value"="Closed loop") -> ("changed or first call?"=w973:bool)
    n725 = case shown="True" "Closed loop" {
      tunnel: w994 -> [_ w1057]
      tunnel: w989 -> [_ w1047]
      tunnel: w979 -> [_ w1075]
      tunnel: "table input switch" -> [_ w1074]
      tunnel: "Thrust Collum" -> [_ w1071]
      tunnel: "Thrust Row" -> [_ w1070]
      tunnel: "Torque Collum" -> [_ w1069]
      tunnel: "Torque Row" -> [_ w1068]
      tunnel: w973 -> [_ w1052]
      frame False {
      }
      frame True {
        w1042 = 1000
        w1050 = 1000
        w1086 = 1.0  # K_f
        w1085 = 1.0  # K_m
        n726 = case shown="True" w1074 {
          tunnel: w1075 -> [_ w1172]
          tunnel: [w1151 w1159] -> w1058
          tunnel: "Total Desired Thrust [g]" -> [w1151 _]
          tunnel: [w1150 w1154] -> w1048
          tunnel: "Total Desired Torque [Nm]" -> [w1150 _]
          tunnel: w1071 -> [_ w1169]
          tunnel: w1070 -> [_ w1168]
          tunnel: w1069 -> [_ w1166]
          tunnel: w1068 -> [_ w1164]
          frame False {
          }
          frame True {
            n727 = Subtract(x=w1164, y=1) -> (x-y=w1163:dbl)
            n728 = Subtract(x=w1168, y=1) -> (x-y=w1167:dbl)
            n729 = Index Array(array=w1172, index (row) #1=w1168, index (col) #1=w1169, index (row) #2=w1167, index (col) #2=w1169, index (row) #3=w1164, index (col) #3=w1166, index (row) #4=w1163, index (col) #4=w1166) -> (element #1=w1171:string, element #2=w1161:string, element #3=w1162:string, element #4=w1160:string)
            n730 = local write "Total Desired Torque [Nm]"(w1154) -> ()
            n731 = Fract/Exp String To Number(string=w1171) -> (number=w1158:dbl)  [unwired: 3 in, 1 out]
            n732 = Fract/Exp String To Number(string=w1161) -> (number=w1157:dbl)  [unwired: 3 in, 1 out]
            n733 = Fract/Exp String To Number(string=w1162) -> (number=w1156:dbl)  [unwired: 3 in, 1 out]
            n734 = Fract/Exp String To Number(string=w1160) -> (number=w1155:dbl)  [unwired: 3 in, 1 out]
            n735 = flat-sequence {
              tunnel: w1158 -> [w1194]
              tunnel: w1157 -> [w1192]
              tunnel: [w1186] -> w1159
              tunnel: [w1185] -> w1152
              frame #0 {
                w1188 = 1
                n736 = call "Is Value Changed.vim"("value"=w1194) -> ("changed or first call?"=w1195:bool)
                n737 = Subtract(x=w1194, y=w1192) -> (x-y=w1193:dbl)
                n738 = call "Elapsed Time5"("Reset"=w1195) -> ("Elapsed Time (s)"=w1185:dbl)  [unwired: 11 in, 7 out]
                n739 = Divide(x=w1185, y=5) -> (x/y=w1187:dbl)
                n740 = Greater?(x=w1187, y=w1188) -> (0:w1189:bool)
                n741 = Select(t=w1188, s=w1189, f=w1187) -> (s? t:f=w1190:dbl)
                n742 = Multiply(x=w1190, y=w1193) -> (x*y=w1191:dbl)
                n743 = Add(x=w1191, y=w1192) -> (x+y=w1186:dbl)
              }
            }
            n744 = flat-sequence {
              tunnel: w1156 -> [w1182]
              tunnel: w1155 -> [w1180]
              tunnel: [w1174] -> w1154
              tunnel: [w1173] -> w1153
              frame #0 {
                w1176 = 1
                n745 = call "Is Value Changed.vim"("value"=w1182) -> ("changed or first call?"=w1183:bool)
                n746 = Subtract(x=w1182, y=w1180) -> (x-y=w1181:dbl)
                n747 = call "Elapsed Time6"("Reset"=w1183) -> ("Elapsed Time (s)"=w1173:dbl)  [unwired: 11 in, 7 out]
                n748 = Divide(x=w1173, y=5) -> (x/y=w1175:dbl)
                n749 = Greater?(x=w1175, y=w1176) -> (0:w1177:bool)
                n750 = Select(t=w1176, s=w1177, f=w1175) -> (s? t:f=w1178:dbl)
                n751 = Multiply(x=w1178, y=w1181) -> (x*y=w1179:dbl)
                n752 = Add(x=w1179, y=w1180) -> (x+y=w1174:dbl)
              }
            }
            n753 = local write "Total Desired Thrust [g]"(w1159) -> ()
            "Thrust Timer [s]" <- w1152
            "Torque Timer [s]" <- w1153
          }
        }
        n754 = Subtract(x=w1048, y=w1047) -> (x-y=w1066:dbl)
        "Torque error [Nm]" <- w1066
        n755 = Bundle("PID Max"="PID Max", "PID Min"="PID Min") -> ()  [unwired: 1 in, 1 out]
        n756 = Subtract(x=w1058, y=w1057) -> (x-y=w1067:dbl)
        "Thrust error [g]" <- w1067
        n757 = Bundle("PID Max"="PID Max", "PID Min"="PID Min") -> ()  [unwired: 1 in, 1 out]
        n758 = Absolute Value(x=w1067) -> (abs(x)=w1034:dbl)
        n759 = Absolute Value(x=w1066) -> (abs(x)=w1063:dbl)
        n760 = flat-sequence {
          tunnel: "kp_m" -> [w1110]
          tunnel: [w1093] -> w1049
          tunnel: "kd_m" -> [w1107]
          tunnel: [w1101] -> w1039
          tunnel: w1048 -> [w1100]
          tunnel: w1047 -> [w1099]
          tunnel: "ki_m" -> [w1098]
          tunnel: w1049 -> [w1111]
          frame #0 {
            n761 = local read "Torque error_last"() -> (w1092:dbl)
            n762 = Subtract(x=w1100, y=w1099) -> (x-y=w1093:dbl)
            n763 = Multiply(x=w1093, y=w1110) -> (x*y=w1104:dbl)
            n764 = Subtract(x=w1092, y=w1093) -> (x-y=w1109:dbl)
            n765 = Divide(x=w1109, y=0.005) -> (x/y=w1096:dbl)
            n766 = call "saturate.vi"("Lower limit"=-1.0, "In"=w1096, "Upper Limit"=1.0) -> ("Out"=w1094:dbl)  [unwired: 8 in]
            "Torque error_d" <- w1094
            n767 = Multiply(x=w1094, y=w1107) -> (x*y=w1103:dbl)
            n768 = local read "Torque error_i"() -> (w1106:dbl)
            n769 = Add(x=w1104, y=w1103) -> (x+y=w1102:dbl)
            n770 = Multiply(x=w1106, y=w1098) -> (x*y=w1105:dbl)
            n771 = Add(x=w1102, y=w1105) -> (x+y=w1101:dbl)
          }
          frame #1 {
            n772 = local read "Torque error_i"() -> (w1118:dbl)
            n773 = Multiply(x=0.005, y=w1111) -> (x*y=w1112:dbl)
            n774 = Add(x=w1112, y=w1118) -> (x+y=w1114:dbl)
            n775 = call "saturate.vi"("Lower limit"=-10, "In"=w1114, "Upper Limit"=10) -> ("Out"=→"Torque error_i":dbl)  [unwired: 8 in]
            "Torque error_last" <- w1111
          }
        }
        n776 = flat-sequence {
          tunnel: w1058 -> [w1126]
          tunnel: w1057 -> [w1138]
          tunnel: "kp_t" -> [w1137]
          tunnel: [w1121] -> w1055
          tunnel: "kd_t" -> [w1134]
          tunnel: "ki_t" -> [w1132]
          tunnel: [w1127] -> w1031
          tunnel: w1055 -> [w1139]
          frame #0 {
            n777 = local read "Thrust error_last"() -> (w1120:dbl)
            n778 = Subtract(x=w1126, y=w1138) -> (x-y=w1121:dbl)
            n779 = Multiply(x=w1121, y=w1137) -> (x*y=w1130:dbl)
            n780 = Subtract(x=w1120, y=w1121) -> (x-y=w1136:dbl)
            n781 = Divide(x=w1136, y=0.005) -> (x/y=w1123:dbl)
            n782 = call "saturate.vi"("Lower limit"=-50.0, "In"=w1123, "Upper Limit"=50.0) -> ("Out"=w1125:dbl)  [unwired: 8 in]
            "Thrust error_d" <- w1125
            n783 = Multiply(x=w1125, y=w1134) -> (x*y=w1129:dbl)
            n784 = local read "Thrust error_i"() -> (w1133:dbl)
            n785 = Add(x=w1130, y=w1129) -> (x+y=w1128:dbl)
            n786 = Multiply(x=w1133, y=w1132) -> (x*y=w1131:dbl)
            n787 = Add(x=w1128, y=w1131) -> (x+y=w1127:dbl)
          }
          frame #1 {
            n788 = local read "Thrust error_i"() -> (w1146:dbl)
            n789 = Multiply(x=0.005, y=w1139) -> (x*y=w1140:dbl)
            n790 = Add(x=w1140, y=w1146) -> (x+y=w1142:dbl)
            n791 = call "saturate.vi"("Lower limit"=-10000, "In"=w1142, "Upper Limit"=10000) -> ("Out"=→"Thrust error_i":dbl)  [unwired: 8 in]
            "Thrust error_last" <- w1139
          }
        }
        n792 = Less?(x=w1034, y="Thrust tolerance [g]") -> (x < y?=w1062:bool)
        n793 = Less?(x=w1063, y="Torque tolerance [Nm]") -> (x < y?=w1061:bool)
        n794 = And(x=w1062, y=w1061) -> (x .and. y?=w1060:bool)
        n795 = Less?(x=w1034, y=100.0) -> (x < y?=w1032:bool)
        n796 = case shown="True" w1060 {
          frame False {
          }
          frame True {
            n797 = local read "Time under tolerance"() -> (w1149:dbl)
            n798 = Add(x=w1149, y=0.005) -> (x+y=→"Time under tolerance":dbl)
          }
        }
        n799 = local read "Thrust PID out"() -> (w1028:dbl)
        n800 = Greater?(x=w1031, y=w1050) -> (0:w1051:bool)
        n801 = Greater?(x=w1039, y=w1042) -> (0:w1043:bool)
        n802 = Select(t=w1050, s=w1051, f=w1031) -> (s? t:f=w1029:dbl)
        n803 = Select(t=w1042, s=w1043, f=w1039) -> (s? t:f=w1030:dbl)
        "Torque PID out" <- w1030
        n804 = case shown="True" w1032 {
          tunnel: w1029 -> [w1087 _]
          frame False {
            "Thrust PID out" <- w1087
          }
          frame True {
            n805 = local read "Thrust error [g]"() -> (w1088:dbl)
            n806 = local read "Thrust PID out"() -> (w1091:dbl)
            n807 = Sign(1:w1088) -> (0:w1090:dbl)
            n808 = Add(x=w1091, y=w1090) -> (x+y=w1089:dbl)
            n809 = local write "Thrust PID out"(w1089) -> ()
          }
        }
        n810 = Multiply(x=w1028, y=w1086) -> (x*y=w1084:dbl)
        n811 = Multiply(x=w1085, y=w1030) -> (x*y=w1083:dbl)
        n812 = case shown="True" w1052 {
          frame False {
          }
          frame True {
            w1119 = 0.0
            n813 = local write "Thrust PID out"(w1119) -> ()
            n814 = local write "Torque PID out"(w1119) -> ()
            n815 = local write "Torque error_i"(w1119) -> ()
            n816 = local write "Thrust error_i"(w1119) -> ()
          }
        }
        n817 = Subtract(x=w1084, y=w1083) -> (x-y=w1081:dbl)
        n818 = Add(x=w1084, y=w1083) -> (x+y=w1079:dbl)
        n819 = Add(x=w1081, y=1000.0 ("K_mr")) -> (x+y=w1077:dbl)
        n820 = Add(x=w1079, y=1000.0 ("K_mr")) -> (x+y=w1036:dbl)
        n821 = call "saturate.vi"("Lower limit"=1050.0, "In"=w1077, "Upper Limit"=1980.0) -> ("Out"=→"Closed Loop Left output":dbl)  [unwired: 8 in]
        n822 = call "saturate.vi"("Lower limit"=1050.0, "In"=w1036, "Upper Limit"=1980.0) -> ("Out"=→"Closed Loop Right output":dbl)  [unwired: 8 in]
      }
    }
  }
